vi "Autonomous Independent.vi"() -> ()   [LabVIEW 2017]
doc: "This VI is called when autonomous begins, and will automatically be terminated when autonomous ends. You can carry out timed or sensor driven robot movement independently without needing to return to the caller."
uses:
  <vilib>/Rock Robotics/WPI/DriverStation/WPI_DriverStationRobotMode2.ctl
  <vilib>/Rock Robotics/WPI/ThirdParty/Phoenix-LabVIEW/Motor Controller/Controls/CTRE_Phoenix_MotorControl_ControlMode.ctl
  <vilib>/Rock Robotics/WPI/Utilities/WPI_GetSetVariantRefNum.vi
  <vilib>/Rock Robotics/Network Tables/NT Read String.vi
  <vilib>/Rock Robotics/Network Tables/NT Write Numeric Array.vi
  <vilib>/Rock Robotics/Network Tables/NT Read Number.vi
  <vilib>/Rock Robotics/Network Tables/NT Write String.vi
  Robot Global Data.vi
  <vilib>/Rock Robotics/Network Tables/NT Write Number.vi
  navx-mxp/labview/navX Library v2/navX Library v2.lvlib
panel:
  out "Game Specific Data":string
  # "Be sure to right-click and choose Data Operations>>Make Current Value default if you want to save the array values with the VI"
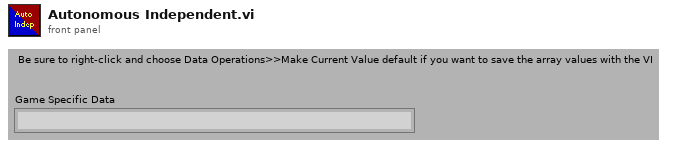
[diagram p1: front panel]
types:
  T1 = typedef "navX Library v2.lvlib/Z900_navX_DeviceTypeDef.ctl" = cluster{"Interface":cluster{"Protocol":T2, "Update Rate (4Hz-100Hz)":u8, "navX Open TypeDef":variant}, "Notify Packet":refnum<notifier>, "Loop VI Refnum":refnum<vi>, "Ready to Close Occurrence Refnum":refnum<k4>}
  T2 = typedef "navX Library v2.lvlib/Z900_navX_ProtocolTypeDef.ctl" = enum16{"SERIAL", "I2C", "SPI"}
  T3 = typedef "WPI_DriverStationRobotMode2.ctl" = enum16{"Autonomous Disabled", "Autonomous Enabled", "Teleop Disabled", "Teleop Enabled", "Disconnected", "Finish", "Test Disabled", "Test Enabled", "Emergency Stopped"}
  T4 = cluster{"Yaw":dbl, "Roll":dbl, "Pitch":dbl, "Heading":dbl, "Fused Heading":dbl}
  T5 = typedef "WPI_GyroDevRef.ctl" = cluster{"DevStatus":errorcluster, "Analog Channel":T6, "Gain (VoltsPerDegree/Second)":dbl, "Gyro Type":enum16{"Analog", "XRS450"}, "Handle":i32, "SPI Bus":T7, "Device Found":bool, "Sample Rate":dbl, "Calibrate On Open":bool, "Offset":dbl}
  T6 = typedef "FPGA_AIChannel.ctl" = enum8{"AI 0", "AI 1", "AI 2", "AI 3", "AI MXP 0", "AI MXP 1", "AI MXP 2", "AI MXP 3", "Invalid"}
  T7 = typedef "spi_bus.ctl" = enum16{"SPI On-Board, CS0", "SPI On-Board, CS1", "SPI On-Board, CS2", "SPI On-Board, CS3", "SPI MXP", "Invalid"}
  T8 = typedef "WPI_JoystickDevRef.ctl" = cluster{"Device":T9}
  T9 = typedef "WPI_JoystickDeviceEnum.ctl" = enum16{"USB 0", "USB 1", "USB 2", "USB 3", "USB 4", "USB 5"}
  T10 = typedef "CTRE_Phoenix_MotorControl_ControlMode.ctl" = u16
  T11 = typedef "WPI_MotorControlDeviceRef.ctl" = cluster{"DeviceStatus":errorcluster, "Type":T12, "PWM":cluster{"PWM Channel":T13, "DeadBand":T14}, "CAN":cluster{"Device Number":u8, "SetOutput VI Ref":variant, "GetOutput VI Ref":variant, "Enable VI Ref":variant, "Disable VI Ref":variant, "Data":variant}, "Invert":bool, "DIO PWM":cluster{"PWM \"Enable\" Channel":T13, "DIOChannel":T15, "PWM Rate":dbl}}
  T12 = typedef "WPI_MotorControlType.ctl" = enum16{"PWM", "CAN", "DIO PWM"}
  T13 = typedef "FPGA_DIOPWMChannel.ctl" = enum8{"PWM 0", "PWM 1", "PWM 2", "PWM 3", "PWM 4", "PWM 5", "PWM 6", "PWM 7", "PWM 8", "PWM 9", "PWM MXP 0", "PWM MXP 1", "PWM MXP 2", "PWM MXP 3", "PWM MXP 4", "PWM MXP 5", "PWM MXP 6", "PWM MXP 7", "PWM MXP 8", "PWM MXP 9", "Invalid"}
  T14 = typedef "WPI_PWMDeadband.ctl" = cluster{"Name":string, "maxPositivePwm":i32, "minPositivePwm":i32, "centerPwm":i32, "maxNegativePwm":i32, "minNegativePwm":i32, "angularRange":u16}
  T15 = typedef "FPGA_DIOChannel.ctl" = enum8{"DIO 0", "DIO 1", "DIO 2", "DIO 3", "DIO 4", "DIO 5", "DIO 6", "DIO 7", "DIO 8", "DIO 9", "DIO MXP 0", "DIO MXP 1", "DIO MXP 2", "DIO MXP 3", "DIO MXP 4", "DIO MXP 5", "DIO MXP 6", "DIO MXP 7", "DIO MXP 8", "DIO MXP 9", "DIO MXP 10", "DIO MXP 11", "DIO MXP 12", "DIO MXP 13", "DIO MXP 14", "DIO MXP 15", "SPI Port CS1", "SPI Port CS2", "SPI Port CS3", "SPI Port MISO", "SPI Port MOSI", "Invalid"}
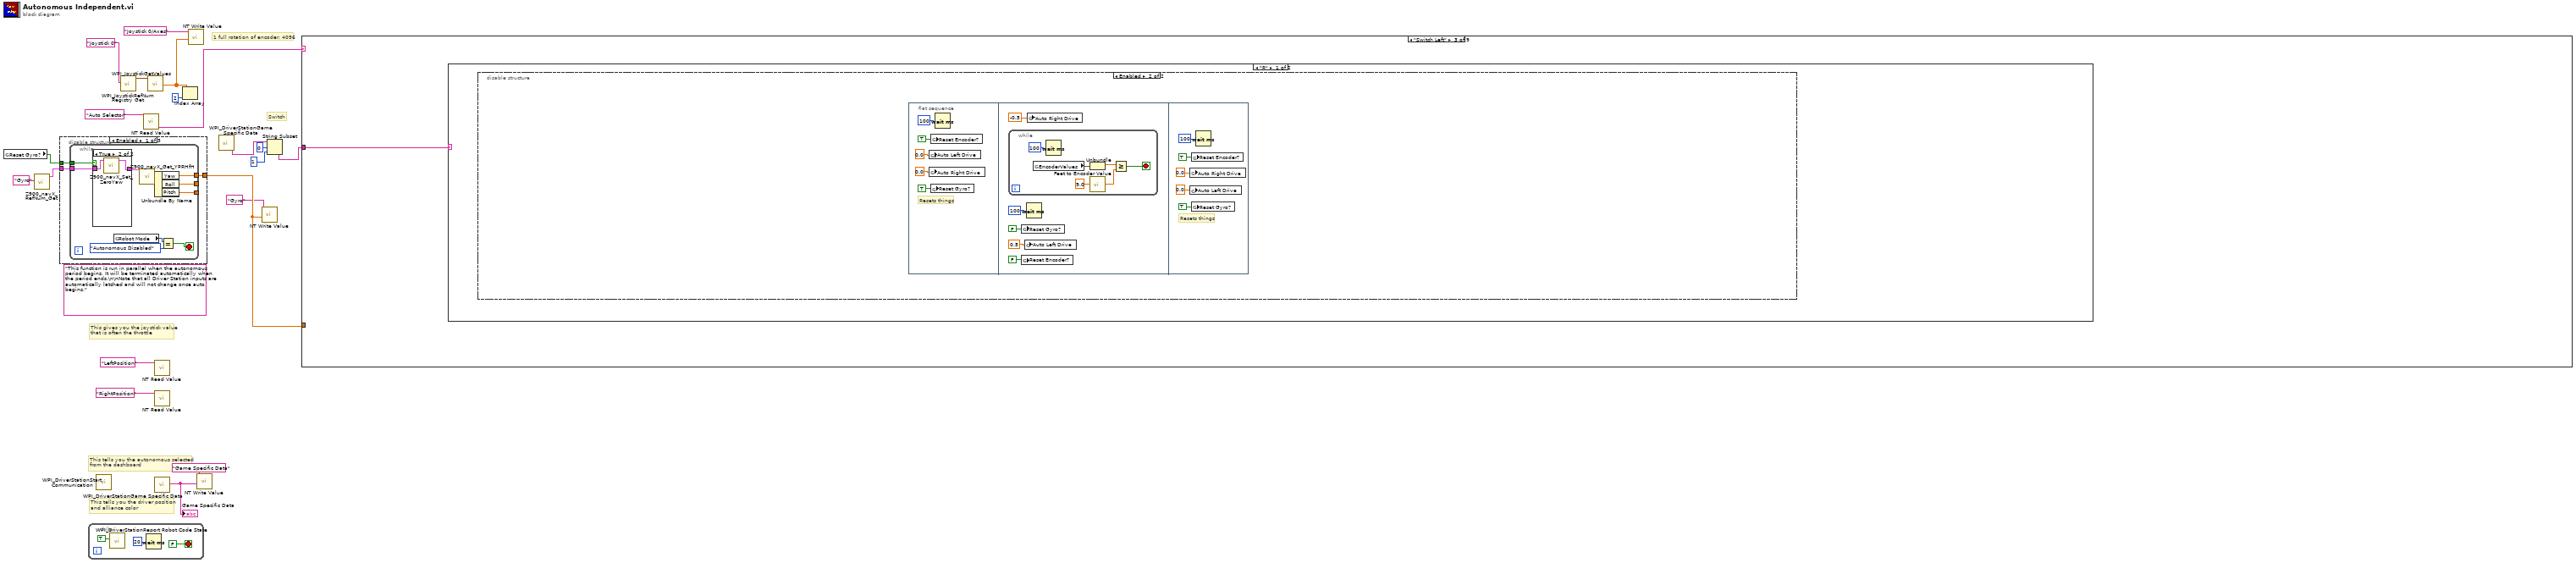
[diagram p0: block diagram]
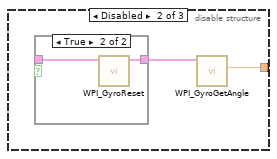
[diagram p3: hidden frame]
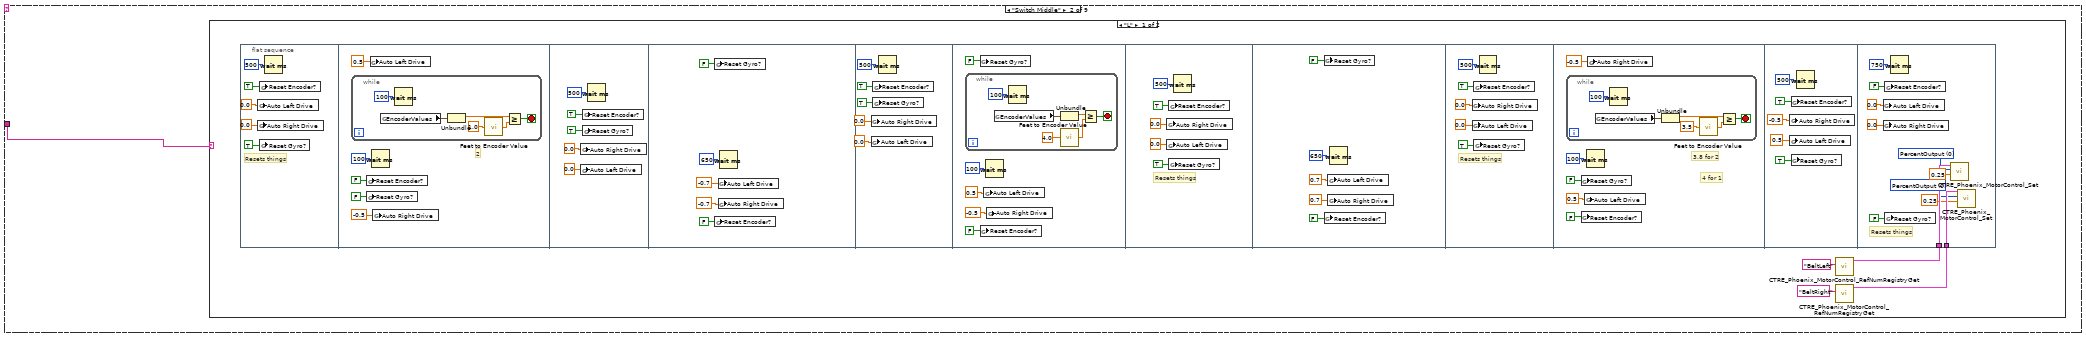
[diagram p7: hidden frame]
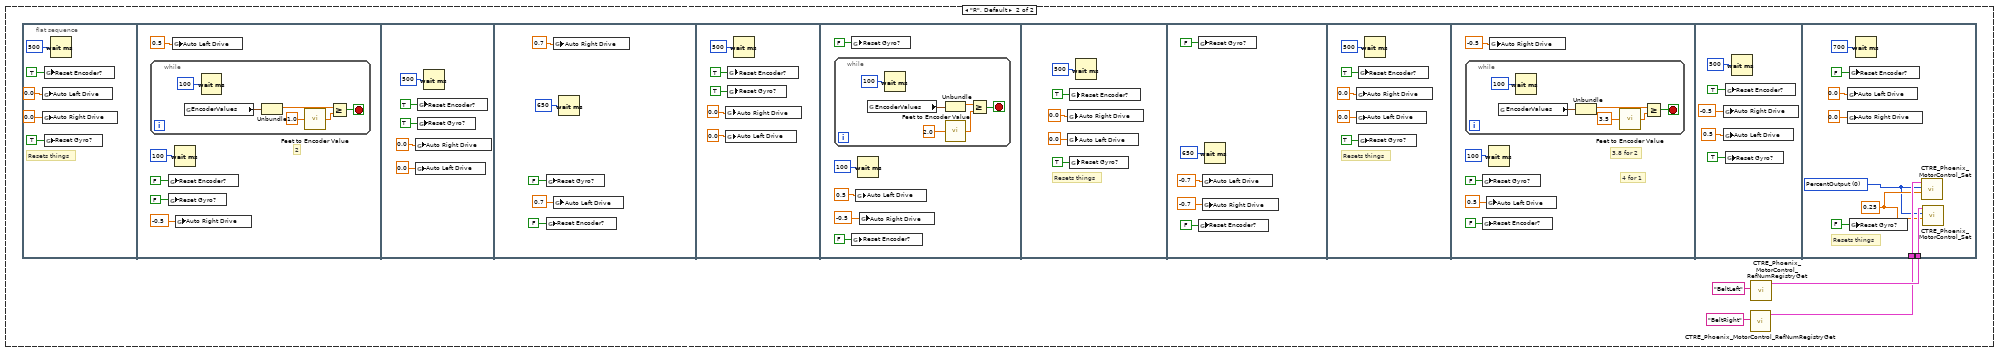
[diagram p8: hidden frame]
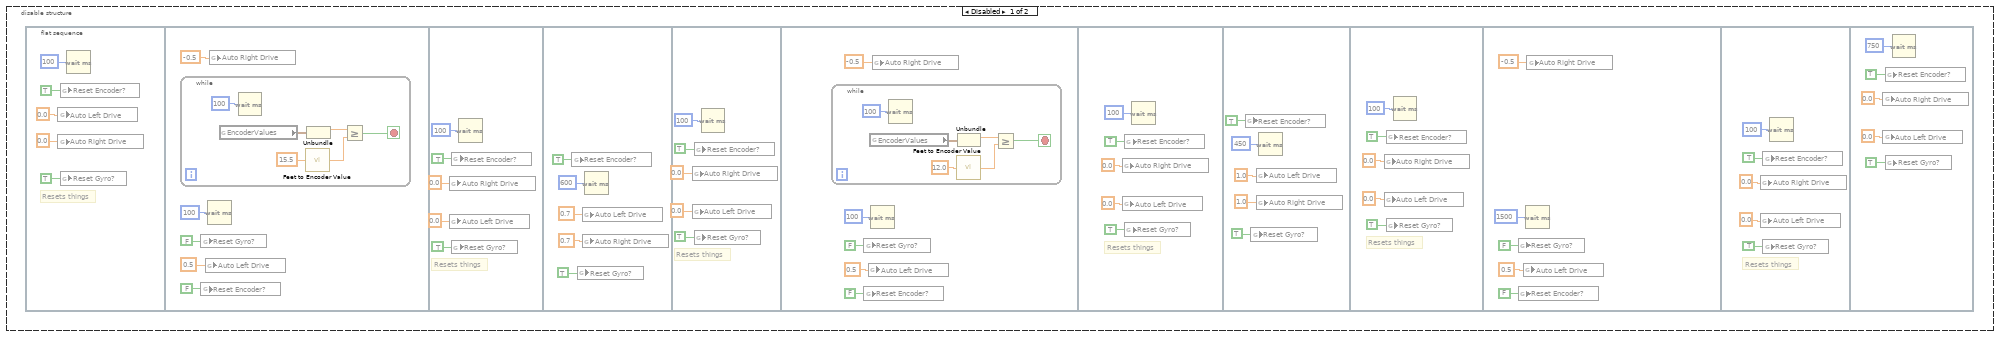
[diagram p9: hidden frame]
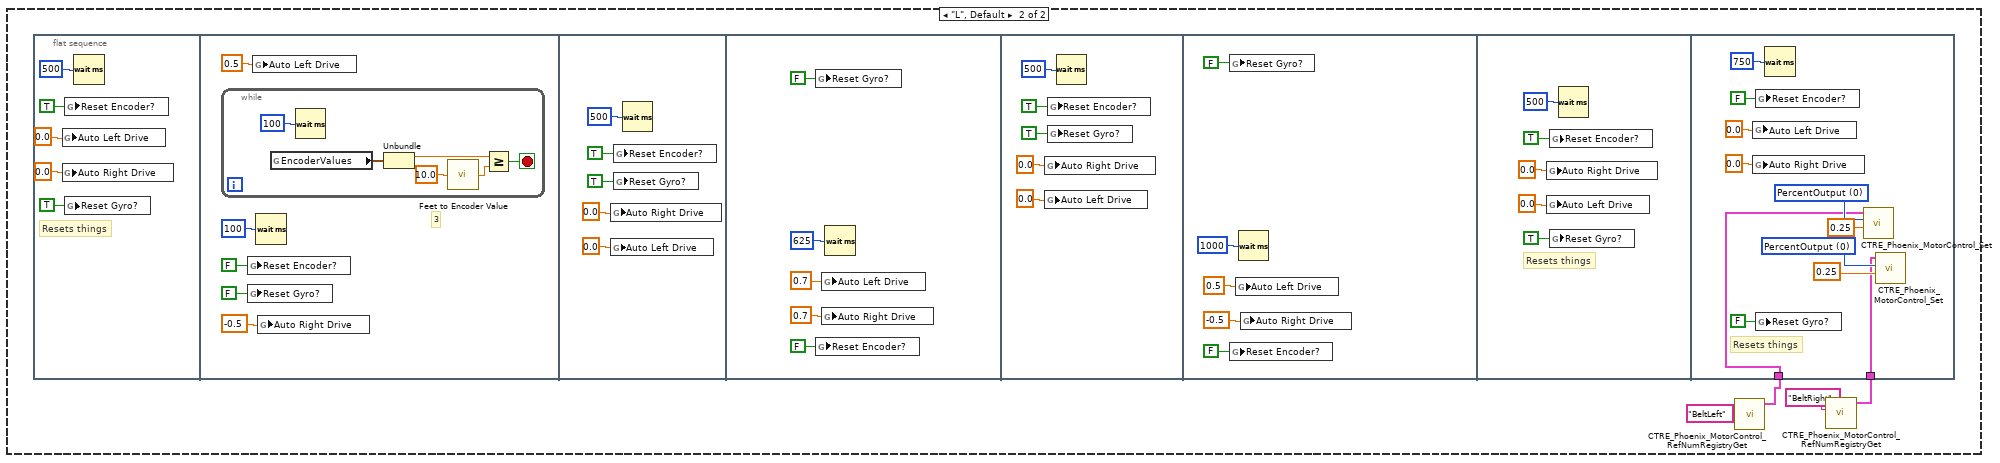
[diagram p10: hidden frame]
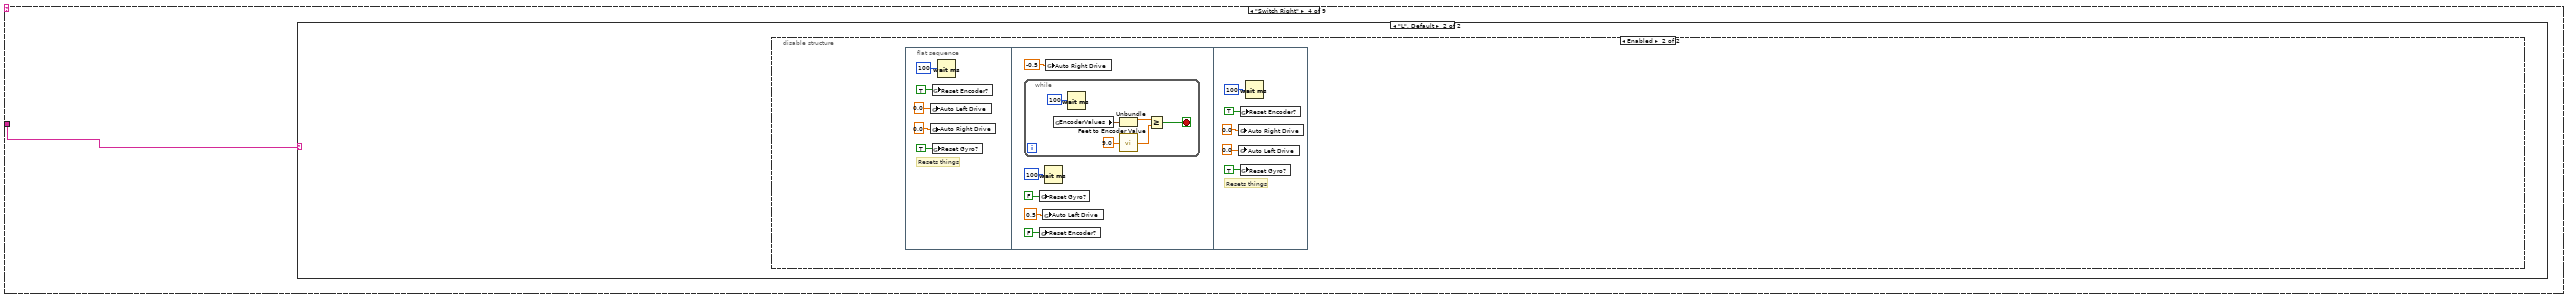
[diagram p11: hidden frame]
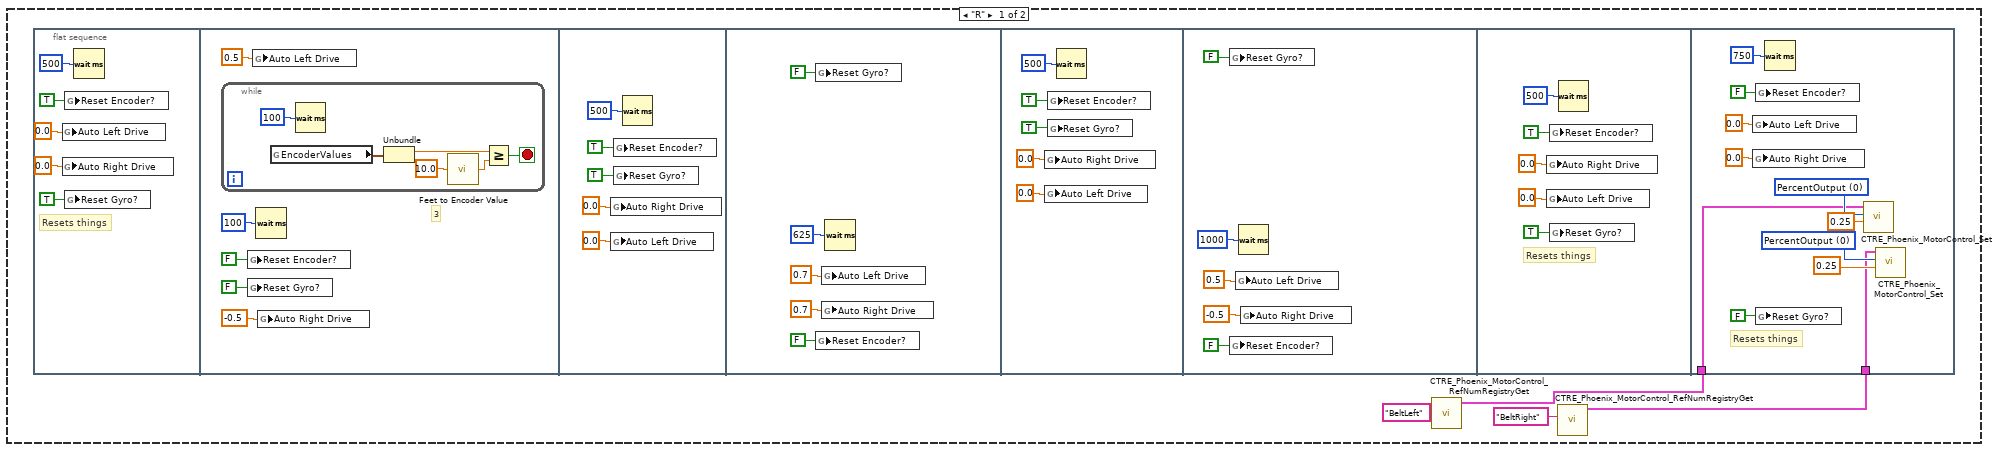
[diagram p12: hidden frame]
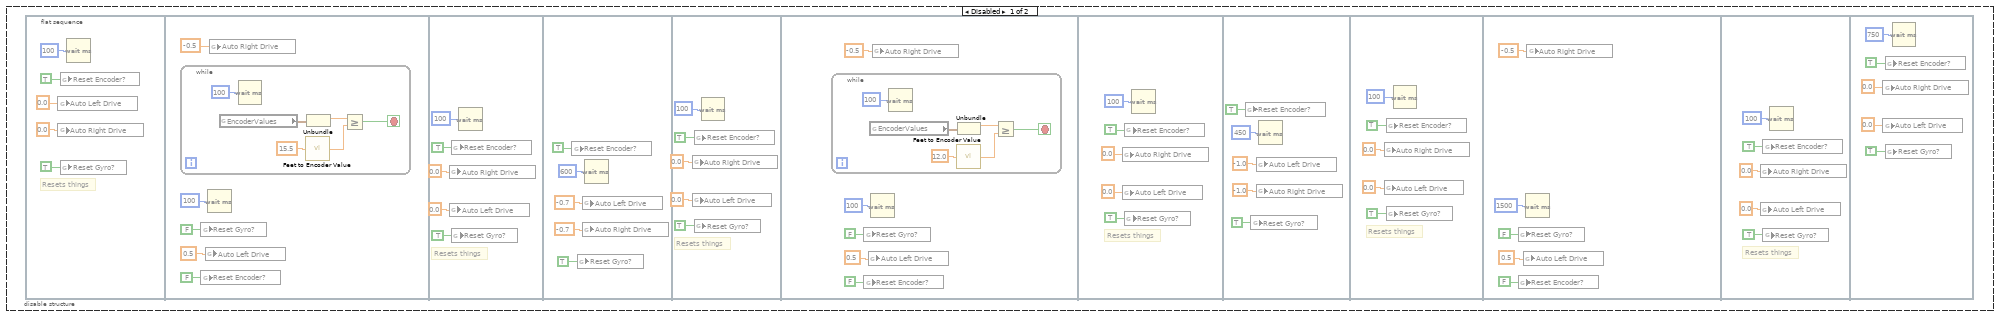
[diagram p13: hidden frame]
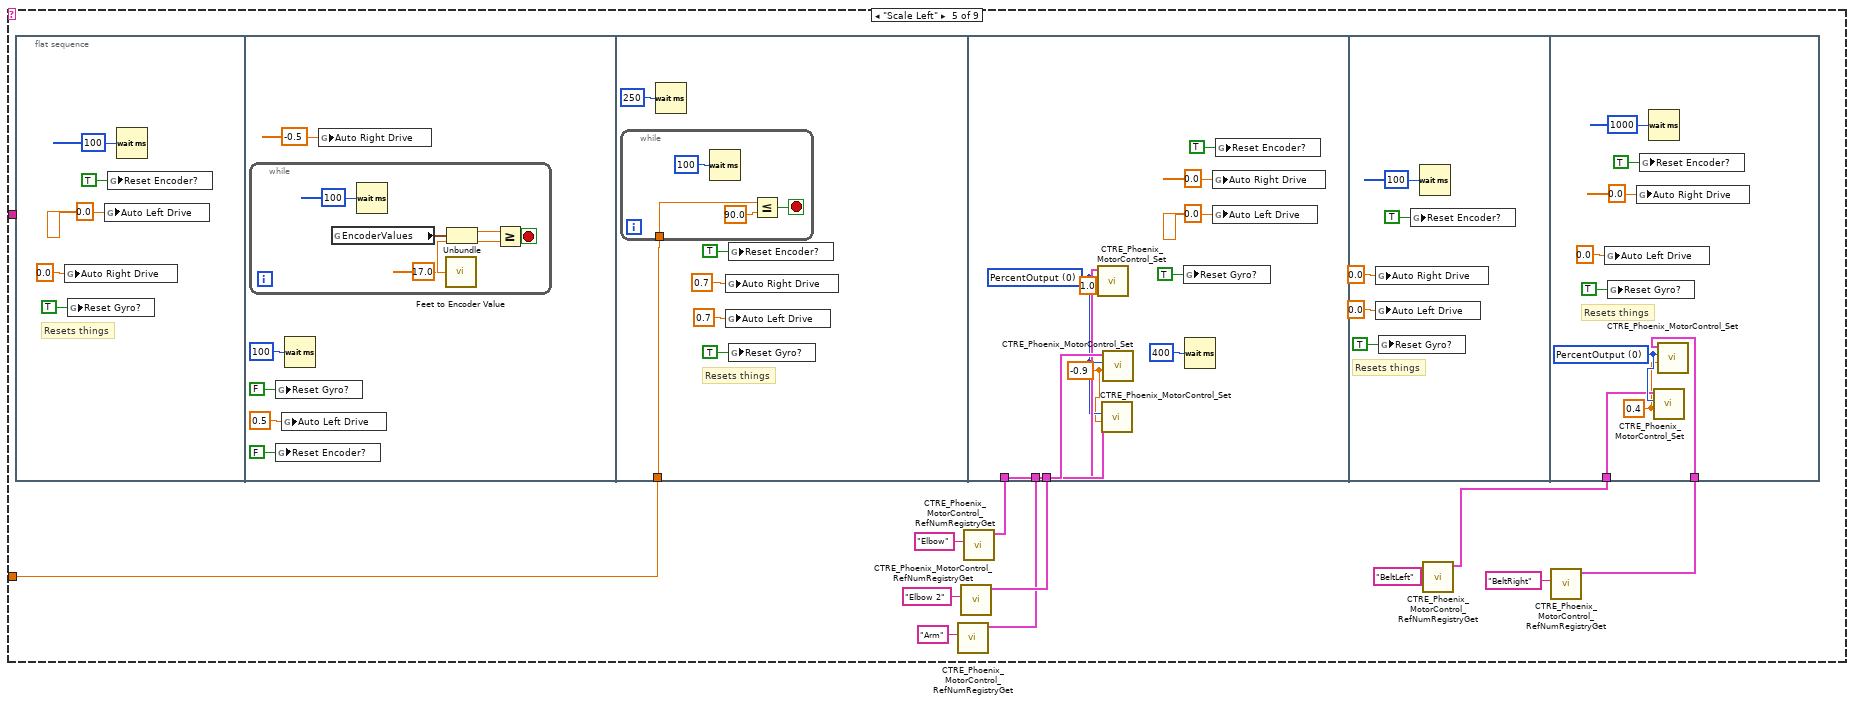
[diagram p14: hidden frame]
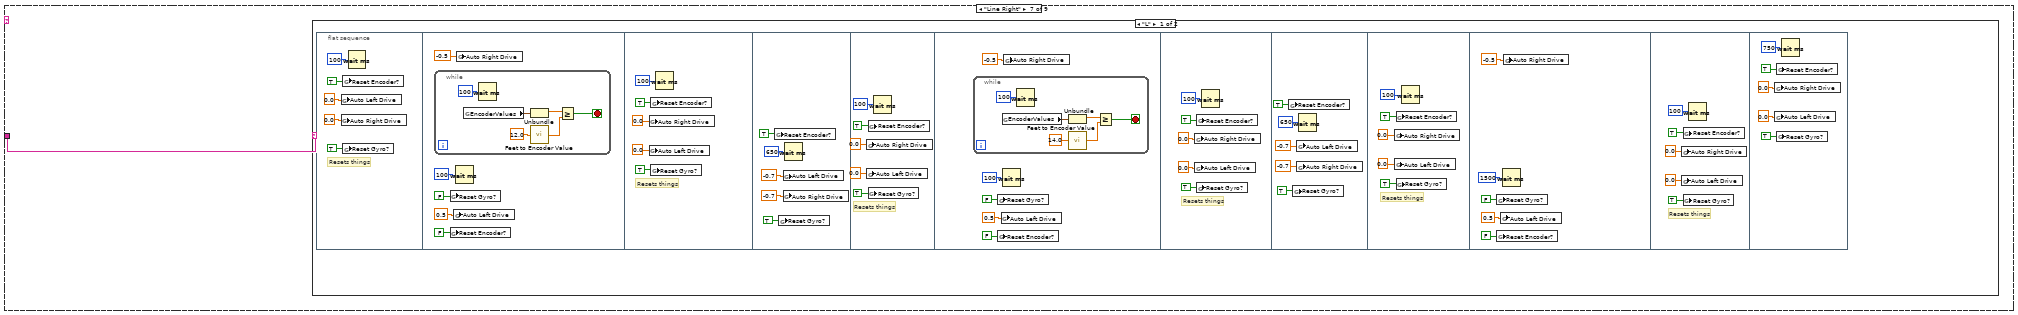
[diagram p16: hidden frame]
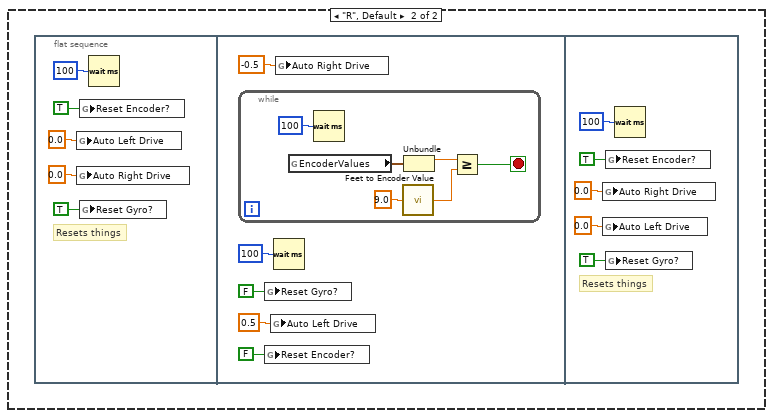
[diagram p17: hidden frame]
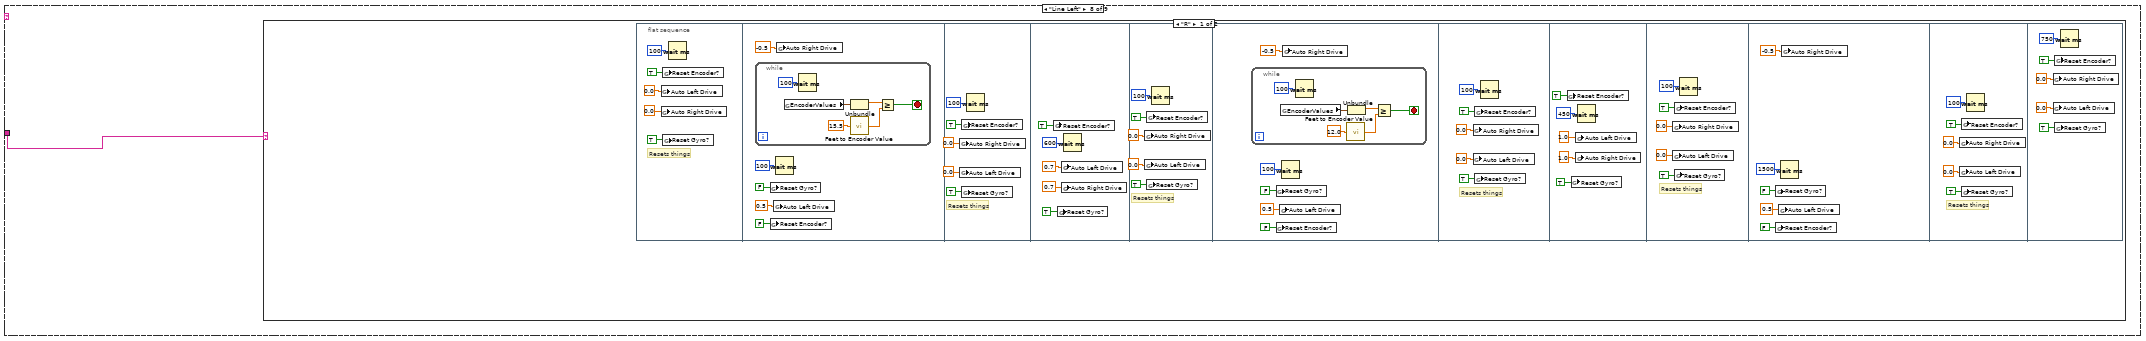
[diagram p18: hidden frame]
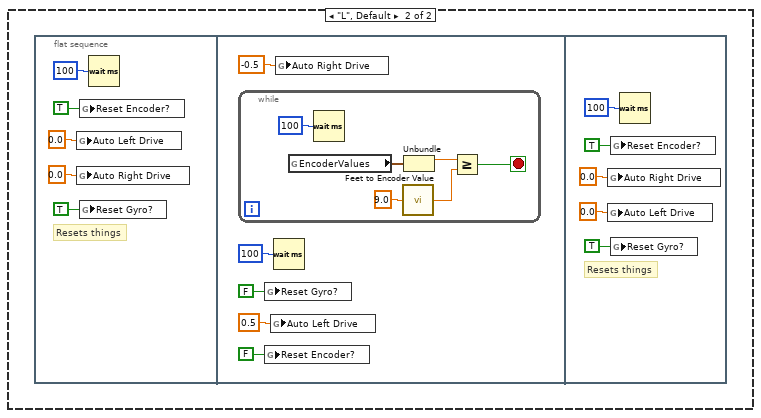
[diagram p19: hidden frame]
diagram:
  (unwired) "This function is run in parallel when the autonomous period begins. It will be terminated automatically when the period ends.\n\nNote that all Driver Station inputs are automatically latched and will not change once auto begins."
  # "Switch"
  # "1 full rotation of encoder: 4096"
  # "This tells you the autonomous selected\nfrom the dashboard"
  # "This gives you the joystick value\nthat is often the throttle"
  # "This tells you the driver position\nand alliance color"
  n1 = global read "Robot Global Data.vi" "Reset Gyro?"() -> (w3:bool)
  n2 = call "Z900_navX_RefNum_Get.vi"("refnum name"="Gyro") -> ("navX Device"=w2:T1)  [unwired: 9 in, 1 out]
  n3 = disable-structure shown="Enabled" {
    disable-tunnel: [w23 w37 _] -> w5
    disable-tunnel: w3 -> [w22 _ _]
    disable-tunnel: w2 -> [w21 _ _]
    frame Enabled {
      n4 = while {
        tunnel: [w27] -> w23
        tunnel: w22 -> [w30]
        tunnel: w21 -> [w26]
        tunnel: [w25] -> _
        tunnel: [w24] -> _
        stop <- w31 stop-if-true
        n5 = case shown="True" w30 {
          tunnel: [w34 w36] -> w29
          tunnel: w26 -> [w34 w35]
          frame False {
          }
          frame True {
            n6 = call "Z900_navX_Set_ZeroYaw.vi"("navX Device"=w35) -> ("navX Device"=w36:T1)  [unwired: 9 in, 1 out]
          }
        }
        n7 = global read "Robot Global Data.vi" "Robot Mode"() -> (w33:T3)
        n8 = call "Z900_navX_Get_YPRHfH.vi"("navX Device"=w29) -> ("YRPHfH"=w28:T4)  [unwired: 7 in, 3 out]
        n9 = Unbundle By Name(w28) -> ("Yaw"=w27:dbl, "Roll"=w25:dbl, "Pitch"=w24:dbl)
        n10 = Equal?(x=w33, y=WPI_DriverStationRobotMode2."Autonomous Disabled") -> (x = y?=w31:bool)
      }
    }
    frame Disabled {
      n11 = case shown="True" {
        selector: _ -> [_ _]
        tunnel: _ -> [w39 w41]
        tunnel: [w39 w40] -> w38
        frame False {
        }
        frame True {
          n12 = call <vilib>:"WPI_GyroReset.vi"("GyroDevRef"=w41) -> ("GyroDevRef"=w40:T5)  [unwired: 9 in, 1 out]
        }
      }
      n13 = call <vilib>:"WPI_GyroGetAngle.vi"("GyroDevRef"=w38) -> ("Angle"=w37:dbl)  [unwired: 6 in, 4 out]
    }
    frame Disabled {
      # "Everything is off :("
    }
  }
  n14 = while {
    stop <- FALSE stop-if-true
    n15 = call <vilib>:"WPI_DriverStationReport Robot Code State.vi"("Autonomous"=TRUE) -> ()  [unwired: 10 in, 1 out]
    n16 = Wait (ms)(milliseconds to wait=u32 20) -> ()  [unwired: 1 out]
  }
  n17 = call <vilib>:"WPI_DriverStationStart Communication.vi"() -> ()  [unwired: 12 in]
  n18 = call <vilib>:"WPI_JoystickRefNum Registry Get.vi"("refnum name"="Joystick 0") -> ("JoystickDevRef"=w19:T8)  [unwired: 1 in, 9 out]
  n19 = call-poly <vilib>:"NT Read Value.vi"("Name"="Auto Selector") -> ("String"=w17:string)  [unwired: 9 in, 1 out]
  n20 = call <vilib>:"WPI_JoystickGetValues.vi"("JoystickDevRef"=w19) -> ("Axes"=w16:dbl[])  [unwired: 6 in, 4 out]
  n21 = call-poly <vilib>:"NT Read Value.vi"("Name"="RightPosition") -> ()  [unwired: 9 in, 2 out]
  n22 = call <vilib>:"WPI_DriverStationGame Specific Data.vi"() -> ("Game Specific Data"=w12:string)  [unwired: 11 in]
  "Game Specific Data" <- w12
  n23 = call-poly <vilib>:"NT Read Value.vi"("Name"="LeftPosition") -> ()  [unwired: 9 in, 2 out]
  n24 = Index Array(array=w16, index=2) -> ()  [unwired: 1 out]
  n25 = call-poly <vilib>:"NT Write Value.vi"("Numeric Array"=w16, "Name"="Joystick 0/Axes") -> ()  [unwired: 9 in, 1 out]
  n26 = call-poly <vilib>:"NT Write Value.vi"("String"=w12, "Name"="Game Specific Data") -> ()  [unwired: 9 in, 1 out]
  n27 = call <vilib>:"WPI_DriverStationGame Specific Data.vi"() -> ("Game Specific Data"=w7:string)  [unwired: 11 in]
  n28 = call-poly <vilib>:"NT Write Value.vi"("Numeric"=w5, "Name"="Gyro") -> ()  [unwired: 9 in, 1 out]
  n29 = String Subset(string=w7, offset (0)=0, length (rest)=1 ("length (rest)")) -> (substring=w8:string)
  n30 = case shown="\"Switch Left\"" w17 {
    tunnel: w8 -> [_ w45 w220 w370 _ _ w581 w675 _]
    tunnel: w5 -> [_ _ _ _ w520 _ _ _ _]
    frame Default {
      # "You can put your main auto here, or you can right-click on the case and make any\nother frame be the default case."
      # "This is the frame that will execute if no selection is made, or if it is not recognized"
    }
    frame "Switch Middle" {
      n31 = case shown="\"L\"" w45 {
        frame "L" {
          n32 = flat-sequence {
            tunnel: w47 -> [w128]
            tunnel: w46 -> [w127]
            frame #0 {
              # "Resets things"
              n33 = global write "Robot Global Data.vi" "Auto Left Drive"(0.0 ("Auto Left Drive")) -> ()
              n34 = global write "Robot Global Data.vi" "Auto Right Drive"(0.0 ("Auto Right Drive")) -> ()
              n35 = global write "Robot Global Data.vi" "Reset Encoder?"(TRUE ("Reset Encoder?")) -> ()
              n36 = global write "Robot Global Data.vi" "Reset Gyro?"(TRUE ("Reset Gyro?")) -> ()
              n37 = Wait (ms)(milliseconds to wait=u32 500) -> ()  [unwired: 1 out]
            }
            frame #1 {
              # "2"
              n38 = while {
                stop <- w60 stop-if-true
                n39 = global read "Robot Global Data.vi" "EncoderValues"() -> (w65:cluster{"EncoderLeft":dbl, "EncoderRight":dbl})
                n40 = Wait (ms)(milliseconds to wait=u32 100) -> ()  [unwired: 1 out]
                n41 = Unbundle(w65) -> ("EncoderLeft"=w64:dbl)  [unwired: 1 out]
                n42 = call "Feet to Encoder Value.vi"("Feet"=1.0) -> ("Encoder Value"=w63:dbl)
                n43 = Greater Or Equal?(x=w64, y=w63) -> (x >= y?=w60:bool)
              }
              n44 = global write "Robot Global Data.vi" "Reset Encoder?"(FALSE ("Reset Encoder?")) -> ()
              n45 = global write "Robot Global Data.vi" "Reset Gyro?"(FALSE ("Reset Gyro?")) -> ()
              n46 = global write "Robot Global Data.vi" "Auto Left Drive"(0.5 ("Auto Left Drive")) -> ()
              n47 = Wait (ms)(milliseconds to wait=u32 100) -> ()  [unwired: 1 out]
              n48 = global write "Robot Global Data.vi" "Auto Right Drive"(-0.5 ("Auto Right Drive")) -> ()
            }
            frame #2 {
              n49 = global write "Robot Global Data.vi" "Auto Right Drive"(0.0 ("Auto Right Drive")) -> ()
              n50 = global write "Robot Global Data.vi" "Auto Left Drive"(0.0 ("Auto Left Drive")) -> ()
              n51 = global write "Robot Global Data.vi" "Reset Encoder?"(TRUE ("Reset Encoder?")) -> ()
              n52 = global write "Robot Global Data.vi" "Reset Gyro?"(TRUE ("Reset Gyro?")) -> ()
              n53 = Wait (ms)(milliseconds to wait=u32 500) -> ()  [unwired: 1 out]
            }
            frame #3 {
              n54 = global write "Robot Global Data.vi" "Reset Gyro?"(FALSE ("Reset Gyro?")) -> ()
              n55 = global write "Robot Global Data.vi" "Reset Encoder?"(FALSE ("Reset Encoder?")) -> ()
              n56 = global write "Robot Global Data.vi" "Auto Left Drive"(-0.7 ("Auto Left Drive")) -> ()
              n57 = global write "Robot Global Data.vi" "Auto Right Drive"(-0.7 ("Auto Right Drive")) -> ()
              n58 = Wait (ms)(milliseconds to wait=u32 650) -> ()  [unwired: 1 out]
            }
            frame #4 {
              n59 = global write "Robot Global Data.vi" "Auto Right Drive"(0.0 ("Auto Right Drive")) -> ()
              n60 = global write "Robot Global Data.vi" "Auto Left Drive"(0.0 ("Auto Left Drive")) -> ()
              n61 = global write "Robot Global Data.vi" "Reset Encoder?"(TRUE ("Reset Encoder?")) -> ()
              n62 = global write "Robot Global Data.vi" "Reset Gyro?"(TRUE ("Reset Gyro?")) -> ()
              n63 = Wait (ms)(milliseconds to wait=u32 500) -> ()  [unwired: 1 out]
            }
            frame #5 {
              n64 = while {
                stop <- w86 stop-if-true
                n65 = global read "Robot Global Data.vi" "EncoderValues"() -> (w91:cluster{"EncoderLeft":dbl, "EncoderRight":dbl})
                n66 = Wait (ms)(milliseconds to wait=u32 100) -> ()  [unwired: 1 out]
                n67 = Unbundle(w91) -> ("EncoderLeft"=w90:dbl)  [unwired: 1 out]
                n68 = call "Feet to Encoder Value.vi"("Feet"=4.0) -> ("Encoder Value"=w89:dbl)
                n69 = Greater Or Equal?(x=w90, y=w89) -> (x >= y?=w86:bool)
              }
              n70 = global write "Robot Global Data.vi" "Reset Gyro?"(FALSE ("Reset Gyro?")) -> ()
              n71 = global write "Robot Global Data.vi" "Reset Encoder?"(FALSE ("Reset Encoder?")) -> ()
              n72 = global write "Robot Global Data.vi" "Auto Left Drive"(0.5 ("Auto Left Drive")) -> ()
              n73 = Wait (ms)(milliseconds to wait=u32 100) -> ()  [unwired: 1 out]
              n74 = global write "Robot Global Data.vi" "Auto Right Drive"(-0.5 ("Auto Right Drive")) -> ()
            }
            frame #6 {
              # "Resets things"
              n75 = global write "Robot Global Data.vi" "Auto Right Drive"(0.0 ("Auto Right Drive")) -> ()
              n76 = global write "Robot Global Data.vi" "Auto Left Drive"(0.0 ("Auto Left Drive")) -> ()
              n77 = global write "Robot Global Data.vi" "Reset Encoder?"(TRUE ("Reset Encoder?")) -> ()
              n78 = global write "Robot Global Data.vi" "Reset Gyro?"(TRUE ("Reset Gyro?")) -> ()
              n79 = Wait (ms)(milliseconds to wait=u32 500) -> ()  [unwired: 1 out]
            }
            frame #7 {
              n80 = global write "Robot Global Data.vi" "Reset Gyro?"(FALSE ("Reset Gyro?")) -> ()
              n81 = global write "Robot Global Data.vi" "Reset Encoder?"(FALSE ("Reset Encoder?")) -> ()
              n82 = global write "Robot Global Data.vi" "Auto Left Drive"(0.7 ("Auto Left Drive")) -> ()
              n83 = global write "Robot Global Data.vi" "Auto Right Drive"(0.7 ("Auto Right Drive")) -> ()
              n84 = Wait (ms)(milliseconds to wait=u32 650) -> ()  [unwired: 1 out]
            }
            frame #8 {
              # "Resets things"
              n85 = global write "Robot Global Data.vi" "Auto Right Drive"(0.0 ("Auto Right Drive")) -> ()
              n86 = global write "Robot Global Data.vi" "Auto Left Drive"(0.0 ("Auto Left Drive")) -> ()
              n87 = global write "Robot Global Data.vi" "Reset Encoder?"(TRUE ("Reset Encoder?")) -> ()
              n88 = global write "Robot Global Data.vi" "Reset Gyro?"(TRUE ("Reset Gyro?")) -> ()
              n89 = Wait (ms)(milliseconds to wait=u32 500) -> ()  [unwired: 1 out]
            }
            frame #9 {
              # "4 for 1"
              # "3.8 for 2"
              n90 = while {
                stop <- w112 stop-if-true
                n91 = global read "Robot Global Data.vi" "EncoderValues"() -> (w117:cluster{"EncoderLeft":dbl, "EncoderRight":dbl})
                n92 = Wait (ms)(milliseconds to wait=u32 100) -> ()  [unwired: 1 out]
                n93 = Unbundle(w117) -> ("EncoderLeft"=w116:dbl)  [unwired: 1 out]
                n94 = call "Feet to Encoder Value.vi"("Feet"=3.5) -> ("Encoder Value"=w115:dbl)
                n95 = Greater Or Equal?(x=w116, y=w115) -> (x >= y?=w112:bool)
              }
              n96 = global write "Robot Global Data.vi" "Reset Gyro?"(FALSE ("Reset Gyro?")) -> ()
              n97 = global write "Robot Global Data.vi" "Reset Encoder?"(FALSE ("Reset Encoder?")) -> ()
              n98 = global write "Robot Global Data.vi" "Auto Left Drive"(0.5 ("Auto Left Drive")) -> ()
              n99 = Wait (ms)(milliseconds to wait=u32 100) -> ()  [unwired: 1 out]
              n100 = global write "Robot Global Data.vi" "Auto Right Drive"(-0.5 ("Auto Right Drive")) -> ()
            }
            frame #10 {
              n101 = global write "Robot Global Data.vi" "Auto Right Drive"(-0.5 ("Auto Right Drive")) -> ()
              n102 = global write "Robot Global Data.vi" "Auto Left Drive"(0.5 ("Auto Left Drive")) -> ()
              n103 = global write "Robot Global Data.vi" "Reset Encoder?"(TRUE ("Reset Encoder?")) -> ()
              n104 = global write "Robot Global Data.vi" "Reset Gyro?"(TRUE ("Reset Gyro?")) -> ()
              n105 = Wait (ms)(milliseconds to wait=u32 500) -> ()  [unwired: 1 out]
            }
            frame #11 {
              w125 = T10 0 items=["PercentOutput"=0, "Position"=1, "Velocity"=2, "Current"=3, "Follower"=5, "MotionProfile"=6, "MotionMagic"=7, "MotionMagicArc"=8, "MotionProfileArc"=10, "Disabled"=15] ("Control Mode")
              w126 = T10 0 items=["PercentOutput"=0, "Position"=1, "Velocity"=2, "Current"=3, "Follower"=5, "MotionProfile"=6, "MotionMagic"=7, "MotionMagicArc"=8, "MotionProfileArc"=10, "Disabled"=15] ("Control Mode")
              # "Resets things"
              n106 = global write "Robot Global Data.vi" "Auto Left Drive"(0.0 ("Auto Left Drive")) -> ()
              n107 = global write "Robot Global Data.vi" "Auto Right Drive"(0.0 ("Auto Right Drive")) -> ()
              n108 = global write "Robot Global Data.vi" "Reset Encoder?"(FALSE ("Reset Encoder?")) -> ()
              n109 = global write "Robot Global Data.vi" "Reset Gyro?"(FALSE ("Reset Gyro?")) -> ()
              n110 = Wait (ms)(milliseconds to wait=u32 750) -> ()  [unwired: 1 out]
              n111 = call <vilib>:"CTRE_Phoenix_MotorControl_Set.vi"("Output"=0.25, "Control Mode"=w126, "PhoenixMotorControlDevRef"=w128) -> ()  [unwired: 7 in, 2 out]
              n112 = call <vilib>:"CTRE_Phoenix_MotorControl_Set.vi"("Output"=0.25, "Control Mode"=w125, "PhoenixMotorControlDevRef"=w127) -> ()  [unwired: 7 in, 2 out]
            }
          }
          n113 = call <vilib>:"CTRE_Phoenix_MotorControl_RefNumRegistryGet.vi"("refnum name"="BeltRight") -> ("PhoenixMotorControlDevRef"=w46:T11)  [unwired: 9 in, 1 out]
          n114 = call <vilib>:"CTRE_Phoenix_MotorControl_RefNumRegistryGet.vi"("refnum name"="BeltLeft") -> ("PhoenixMotorControlDevRef"=w47:T11)  [unwired: 9 in, 1 out]
        }
        frame "R", Default {
          n115 = flat-sequence {
            tunnel: w135 -> [w214]
            tunnel: w134 -> [w213]
            frame #0 {
              # "Resets things"
              n116 = global write "Robot Global Data.vi" "Auto Left Drive"(0.0 ("Auto Left Drive")) -> ()
              n117 = global write "Robot Global Data.vi" "Auto Right Drive"(0.0 ("Auto Right Drive")) -> ()
              n118 = global write "Robot Global Data.vi" "Reset Encoder?"(TRUE ("Reset Encoder?")) -> ()
              n119 = global write "Robot Global Data.vi" "Reset Gyro?"(TRUE ("Reset Gyro?")) -> ()
              n120 = Wait (ms)(milliseconds to wait=u32 500) -> ()  [unwired: 1 out]
            }
            frame #1 {
              # "2"
              n121 = while {
                stop <- w148 stop-if-true
                n122 = global read "Robot Global Data.vi" "EncoderValues"() -> (w153:cluster{"EncoderLeft":dbl, "EncoderRight":dbl})
                n123 = Wait (ms)(milliseconds to wait=u32 100) -> ()  [unwired: 1 out]
                n124 = Unbundle(w153) -> ("EncoderLeft"=w152:dbl)  [unwired: 1 out]
                n125 = call "Feet to Encoder Value.vi"("Feet"=1.0) -> ("Encoder Value"=w151:dbl)
                n126 = Greater Or Equal?(x=w152, y=w151) -> (x >= y?=w148:bool)
              }
              n127 = global write "Robot Global Data.vi" "Reset Encoder?"(FALSE ("Reset Encoder?")) -> ()
              n128 = global write "Robot Global Data.vi" "Reset Gyro?"(FALSE ("Reset Gyro?")) -> ()
              n129 = global write "Robot Global Data.vi" "Auto Left Drive"(0.5 ("Auto Left Drive")) -> ()
              n130 = Wait (ms)(milliseconds to wait=u32 100) -> ()  [unwired: 1 out]
              n131 = global write "Robot Global Data.vi" "Auto Right Drive"(-0.5 ("Auto Right Drive")) -> ()
            }
            frame #2 {
              n132 = global write "Robot Global Data.vi" "Auto Right Drive"(0.0 ("Auto Right Drive")) -> ()
              n133 = global write "Robot Global Data.vi" "Auto Left Drive"(0.0 ("Auto Left Drive")) -> ()
              n134 = global write "Robot Global Data.vi" "Reset Encoder?"(TRUE ("Reset Encoder?")) -> ()
              n135 = global write "Robot Global Data.vi" "Reset Gyro?"(TRUE ("Reset Gyro?")) -> ()
              n136 = Wait (ms)(milliseconds to wait=u32 500) -> ()  [unwired: 1 out]
            }
            frame #3 {
              n137 = global write "Robot Global Data.vi" "Reset Gyro?"(FALSE ("Reset Gyro?")) -> ()
              n138 = global write "Robot Global Data.vi" "Reset Encoder?"(FALSE ("Reset Encoder?")) -> ()
              n139 = global write "Robot Global Data.vi" "Auto Right Drive"(0.7 ("Auto Right Drive")) -> ()
              n140 = global write "Robot Global Data.vi" "Auto Left Drive"(0.7 ("Auto Left Drive")) -> ()
              n141 = Wait (ms)(milliseconds to wait=u32 650) -> ()  [unwired: 1 out]
            }
            frame #4 {
              n142 = global write "Robot Global Data.vi" "Auto Right Drive"(0.0 ("Auto Right Drive")) -> ()
              n143 = global write "Robot Global Data.vi" "Auto Left Drive"(0.0 ("Auto Left Drive")) -> ()
              n144 = global write "Robot Global Data.vi" "Reset Encoder?"(TRUE ("Reset Encoder?")) -> ()
              n145 = global write "Robot Global Data.vi" "Reset Gyro?"(TRUE ("Reset Gyro?")) -> ()
              n146 = Wait (ms)(milliseconds to wait=u32 500) -> ()  [unwired: 1 out]
            }
            frame #5 {
              n147 = while {
                stop <- w174 stop-if-true
                n148 = global read "Robot Global Data.vi" "EncoderValues"() -> (w179:cluster{"EncoderLeft":dbl, "EncoderRight":dbl})
                n149 = Wait (ms)(milliseconds to wait=u32 100) -> ()  [unwired: 1 out]
                n150 = Unbundle(w179) -> ("EncoderLeft"=w178:dbl)  [unwired: 1 out]
                n151 = call "Feet to Encoder Value.vi"("Feet"=2.0) -> ("Encoder Value"=w177:dbl)
                n152 = Greater Or Equal?(x=w178, y=w177) -> (x >= y?=w174:bool)
              }
              n153 = global write "Robot Global Data.vi" "Reset Gyro?"(FALSE ("Reset Gyro?")) -> ()
              n154 = global write "Robot Global Data.vi" "Reset Encoder?"(FALSE ("Reset Encoder?")) -> ()
              n155 = global write "Robot Global Data.vi" "Auto Left Drive"(0.5 ("Auto Left Drive")) -> ()
              n156 = Wait (ms)(milliseconds to wait=u32 100) -> ()  [unwired: 1 out]
              n157 = global write "Robot Global Data.vi" "Auto Right Drive"(-0.5 ("Auto Right Drive")) -> ()
            }
            frame #6 {
              # "Resets things"
              n158 = global write "Robot Global Data.vi" "Auto Right Drive"(0.0 ("Auto Right Drive")) -> ()
              n159 = global write "Robot Global Data.vi" "Auto Left Drive"(0.0 ("Auto Left Drive")) -> ()
              n160 = global write "Robot Global Data.vi" "Reset Encoder?"(TRUE ("Reset Encoder?")) -> ()
              n161 = global write "Robot Global Data.vi" "Reset Gyro?"(TRUE ("Reset Gyro?")) -> ()
              n162 = Wait (ms)(milliseconds to wait=u32 500) -> ()  [unwired: 1 out]
            }
            frame #7 {
              n163 = global write "Robot Global Data.vi" "Reset Gyro?"(FALSE ("Reset Gyro?")) -> ()
              n164 = global write "Robot Global Data.vi" "Reset Encoder?"(FALSE ("Reset Encoder?")) -> ()
              n165 = global write "Robot Global Data.vi" "Auto Left Drive"(-0.7 ("Auto Left Drive")) -> ()
              n166 = global write "Robot Global Data.vi" "Auto Right Drive"(-0.7 ("Auto Right Drive")) -> ()
              n167 = Wait (ms)(milliseconds to wait=u32 650) -> ()  [unwired: 1 out]
            }
            frame #8 {
              # "Resets things"
              n168 = global write "Robot Global Data.vi" "Auto Right Drive"(0.0 ("Auto Right Drive")) -> ()
              n169 = global write "Robot Global Data.vi" "Auto Left Drive"(0.0 ("Auto Left Drive")) -> ()
              n170 = global write "Robot Global Data.vi" "Reset Encoder?"(TRUE ("Reset Encoder?")) -> ()
              n171 = global write "Robot Global Data.vi" "Reset Gyro?"(TRUE ("Reset Gyro?")) -> ()
              n172 = Wait (ms)(milliseconds to wait=u32 500) -> ()  [unwired: 1 out]
            }
            frame #9 {
              # "4 for 1"
              # "3.8 for 2"
              n173 = while {
                stop <- w200 stop-if-true
                n174 = global read "Robot Global Data.vi" "EncoderValues"() -> (w205:cluster{"EncoderLeft":dbl, "EncoderRight":dbl})
                n175 = Wait (ms)(milliseconds to wait=u32 100) -> ()  [unwired: 1 out]
                n176 = Unbundle(w205) -> ("EncoderLeft"=w204:dbl)  [unwired: 1 out]
                n177 = call "Feet to Encoder Value.vi"("Feet"=3.5) -> ("Encoder Value"=w203:dbl)
                n178 = Greater Or Equal?(x=w204, y=w203) -> (x >= y?=w200:bool)
              }
              n179 = global write "Robot Global Data.vi" "Reset Gyro?"(FALSE ("Reset Gyro?")) -> ()
              n180 = global write "Robot Global Data.vi" "Reset Encoder?"(FALSE ("Reset Encoder?")) -> ()
              n181 = global write "Robot Global Data.vi" "Auto Left Drive"(0.5 ("Auto Left Drive")) -> ()
              n182 = Wait (ms)(milliseconds to wait=u32 100) -> ()  [unwired: 1 out]
              n183 = global write "Robot Global Data.vi" "Auto Right Drive"(-0.5 ("Auto Right Drive")) -> ()
            }
            frame #10 {
              n184 = global write "Robot Global Data.vi" "Auto Right Drive"(-0.5 ("Auto Right Drive")) -> ()
              n185 = global write "Robot Global Data.vi" "Auto Left Drive"(0.5 ("Auto Left Drive")) -> ()
              n186 = global write "Robot Global Data.vi" "Reset Encoder?"(TRUE ("Reset Encoder?")) -> ()
              n187 = global write "Robot Global Data.vi" "Reset Gyro?"(TRUE ("Reset Gyro?")) -> ()
              n188 = Wait (ms)(milliseconds to wait=u32 500) -> ()  [unwired: 1 out]
            }
            frame #11 {
              w211 = T10 0 items=["PercentOutput"=0, "Position"=1, "Velocity"=2, "Current"=3, "Follower"=5, "MotionProfile"=6, "MotionMagic"=7, "MotionMagicArc"=8, "MotionProfileArc"=10, "Disabled"=15] ("Control Mode")
              w212 = 0.25 ("Output")
              # "Resets things"
              n189 = global write "Robot Global Data.vi" "Auto Left Drive"(0.0 ("Auto Left Drive")) -> ()
              n190 = global write "Robot Global Data.vi" "Auto Right Drive"(0.0 ("Auto Right Drive")) -> ()
              n191 = global write "Robot Global Data.vi" "Reset Encoder?"(FALSE ("Reset Encoder?")) -> ()
              n192 = global write "Robot Global Data.vi" "Reset Gyro?"(FALSE ("Reset Gyro?")) -> ()
              n193 = Wait (ms)(milliseconds to wait=u32 700) -> ()  [unwired: 1 out]
              n194 = call <vilib>:"CTRE_Phoenix_MotorControl_Set.vi"("Output"=w212, "Control Mode"=w211, "PhoenixMotorControlDevRef"=w213) -> ()  [unwired: 7 in, 2 out]
              n195 = call <vilib>:"CTRE_Phoenix_MotorControl_Set.vi"("Output"=w212, "Control Mode"=w211, "PhoenixMotorControlDevRef"=w214) -> ()  [unwired: 7 in, 2 out]
            }
          }
          n196 = call <vilib>:"CTRE_Phoenix_MotorControl_RefNumRegistryGet.vi"("refnum name"="BeltRight") -> ("PhoenixMotorControlDevRef"=w134:T11)  [unwired: 9 in, 1 out]
          n197 = call <vilib>:"CTRE_Phoenix_MotorControl_RefNumRegistryGet.vi"("refnum name"="BeltLeft") -> ("PhoenixMotorControlDevRef"=w135:T11)  [unwired: 9 in, 1 out]
        }
      }
    }
    frame "Switch Left" {
      n198 = case shown="\"R\"" w220 {
        frame "R" {
          n199 = disable-structure shown="Enabled" {
            frame Disabled {
              n200 = flat-sequence {
                frame #0 {
                  # "Resets things"
                  n201 = global write "Robot Global Data.vi" "Auto Left Drive"(0.0 ("Auto Left Drive")) -> ()
                  n202 = global write "Robot Global Data.vi" "Auto Right Drive"(0.0 ("Auto Right Drive")) -> ()
                  n203 = global write "Robot Global Data.vi" "Reset Encoder?"(TRUE ("Reset Encoder?")) -> ()
                  n204 = global write "Robot Global Data.vi" "Reset Gyro?"(TRUE ("Reset Gyro?")) -> ()
                  n205 = Wait (ms)(milliseconds to wait=u32 100) -> ()  [unwired: 1 out]
                }
                frame #1 {
                  n206 = while {
                    stop <- w231 stop-if-true
                    n207 = global read "Robot Global Data.vi" "EncoderValues"() -> (w236:cluster{"EncoderLeft":dbl, "EncoderRight":dbl})
                    n208 = Wait (ms)(milliseconds to wait=u32 100) -> ()  [unwired: 1 out]
                    n209 = call "Feet to Encoder Value.vi"("Feet"=15.5) -> ("Encoder Value"=w234:dbl)
                    n210 = Unbundle(w236) -> ("EncoderLeft"=w235:dbl)  [unwired: 1 out]
                    n211 = Greater Or Equal?(x=w235, y=w234) -> (x >= y?=w231:bool)
                  }
                  n212 = global write "Robot Global Data.vi" "Reset Gyro?"(FALSE ("Reset Gyro?")) -> ()
                  n213 = global write "Robot Global Data.vi" "Reset Encoder?"(FALSE ("Reset Encoder?")) -> ()
                  n214 = global write "Robot Global Data.vi" "Auto Left Drive"(0.5 ("Auto Left Drive")) -> ()
                  n215 = Wait (ms)(milliseconds to wait=u32 100) -> ()  [unwired: 1 out]
                  n216 = global write "Robot Global Data.vi" "Auto Right Drive"(-0.5 ("Auto Right Drive")) -> ()
                }
                frame #2 {
                  # "Resets things"
                  n217 = global write "Robot Global Data.vi" "Auto Right Drive"(0.0 ("Auto Right Drive")) -> ()
                  n218 = global write "Robot Global Data.vi" "Auto Left Drive"(0.0 ("Auto Left Drive")) -> ()
                  n219 = global write "Robot Global Data.vi" "Reset Encoder?"(TRUE ("Reset Encoder?")) -> ()
                  n220 = global write "Robot Global Data.vi" "Reset Gyro?"(TRUE ("Reset Gyro?")) -> ()
                  n221 = Wait (ms)(milliseconds to wait=u32 100) -> ()  [unwired: 1 out]
                }
                frame #3 {
                  n222 = global write "Robot Global Data.vi" "Reset Encoder?"(TRUE ("Reset Encoder?")) -> ()
                  n223 = global write "Robot Global Data.vi" "Reset Gyro?"(TRUE ("Reset Gyro?")) -> ()
                  n224 = global write "Robot Global Data.vi" "Auto Left Drive"(0.7 ("Auto Left Drive")) -> ()
                  n225 = global write "Robot Global Data.vi" "Auto Right Drive"(0.7 ("Auto Right Drive")) -> ()
                  n226 = Wait (ms)(milliseconds to wait=u32 600) -> ()  [unwired: 1 out]
                }
                frame #4 {
                  # "Resets things"
                  n227 = global write "Robot Global Data.vi" "Auto Right Drive"(0.0 ("Auto Right Drive")) -> ()
                  n228 = global write "Robot Global Data.vi" "Auto Left Drive"(0.0 ("Auto Left Drive")) -> ()
                  n229 = global write "Robot Global Data.vi" "Reset Encoder?"(TRUE ("Reset Encoder?")) -> ()
                  n230 = global write "Robot Global Data.vi" "Reset Gyro?"(TRUE ("Reset Gyro?")) -> ()
                  n231 = Wait (ms)(milliseconds to wait=u32 100) -> ()  [unwired: 1 out]
                }
                frame #5 {
                  n232 = while {
                    stop <- w257 stop-if-true
                    n233 = global read "Robot Global Data.vi" "EncoderValues"() -> (w262:cluster{"EncoderLeft":dbl, "EncoderRight":dbl})
                    n234 = Wait (ms)(milliseconds to wait=u32 100) -> ()  [unwired: 1 out]
                    n235 = call "Feet to Encoder Value.vi"("Feet"=12.0) -> ("Encoder Value"=w260:dbl)
                    n236 = Unbundle(w262) -> ("EncoderLeft"=w261:dbl)  [unwired: 1 out]
                    n237 = Greater Or Equal?(x=w261, y=w260) -> (x >= y?=w257:bool)
                  }
                  n238 = global write "Robot Global Data.vi" "Reset Gyro?"(FALSE ("Reset Gyro?")) -> ()
                  n239 = global write "Robot Global Data.vi" "Reset Encoder?"(FALSE ("Reset Encoder?")) -> ()
                  n240 = global write "Robot Global Data.vi" "Auto Left Drive"(0.5 ("Auto Left Drive")) -> ()
                  n241 = Wait (ms)(milliseconds to wait=u32 100) -> ()  [unwired: 1 out]
                  n242 = global write "Robot Global Data.vi" "Auto Right Drive"(-0.5 ("Auto Right Drive")) -> ()
                }
                frame #6 {
                  # "Resets things"
                  n243 = global write "Robot Global Data.vi" "Auto Right Drive"(0.0 ("Auto Right Drive")) -> ()
                  n244 = global write "Robot Global Data.vi" "Auto Left Drive"(0.0 ("Auto Left Drive")) -> ()
                  n245 = global write "Robot Global Data.vi" "Reset Encoder?"(TRUE ("Reset Encoder?")) -> ()
                  n246 = global write "Robot Global Data.vi" "Reset Gyro?"(TRUE ("Reset Gyro?")) -> ()
                  n247 = Wait (ms)(milliseconds to wait=u32 100) -> ()  [unwired: 1 out]
                }
                frame #7 {
                  n248 = global write "Robot Global Data.vi" "Reset Encoder?"(TRUE ("Reset Encoder?")) -> ()
                  n249 = global write "Robot Global Data.vi" "Reset Gyro?"(TRUE ("Reset Gyro?")) -> ()
                  n250 = global write "Robot Global Data.vi" "Auto Left Drive"(1.0 ("Auto Left Drive")) -> ()
                  n251 = global write "Robot Global Data.vi" "Auto Right Drive"(1.0 ("Auto Right Drive")) -> ()
                  n252 = Wait (ms)(milliseconds to wait=u32 450) -> ()  [unwired: 1 out]
                }
                frame #8 {
                  # "Resets things"
                  n253 = global write "Robot Global Data.vi" "Auto Right Drive"(0.0 ("Auto Right Drive")) -> ()
                  n254 = global write "Robot Global Data.vi" "Auto Left Drive"(0.0 ("Auto Left Drive")) -> ()
                  n255 = global write "Robot Global Data.vi" "Reset Encoder?"(TRUE ("Reset Encoder?")) -> ()
                  n256 = global write "Robot Global Data.vi" "Reset Gyro?"(TRUE ("Reset Gyro?")) -> ()
                  n257 = Wait (ms)(milliseconds to wait=u32 100) -> ()  [unwired: 1 out]
                }
                frame #9 {
                  n258 = global write "Robot Global Data.vi" "Reset Gyro?"(FALSE ("Reset Gyro?")) -> ()
                  n259 = global write "Robot Global Data.vi" "Reset Encoder?"(FALSE ("Reset Encoder?")) -> ()
                  n260 = global write "Robot Global Data.vi" "Auto Left Drive"(0.5 ("Auto Left Drive")) -> ()
                  n261 = Wait (ms)(milliseconds to wait=u32 1500) -> ()  [unwired: 1 out]
                  n262 = global write "Robot Global Data.vi" "Auto Right Drive"(-0.5 ("Auto Right Drive")) -> ()
                }
                frame #10 {
                  # "Resets things"
                  n263 = global write "Robot Global Data.vi" "Auto Right Drive"(0.0 ("Auto Right Drive")) -> ()
                  n264 = global write "Robot Global Data.vi" "Auto Left Drive"(0.0 ("Auto Left Drive")) -> ()
                  n265 = global write "Robot Global Data.vi" "Reset Encoder?"(TRUE ("Reset Encoder?")) -> ()
                  n266 = global write "Robot Global Data.vi" "Reset Gyro?"(TRUE ("Reset Gyro?")) -> ()
                  n267 = Wait (ms)(milliseconds to wait=u32 100) -> ()  [unwired: 1 out]
                }
                frame #11 {
                  n268 = global write "Robot Global Data.vi" "Auto Right Drive"(0.0 ("Auto Right Drive")) -> ()
                  n269 = global write "Robot Global Data.vi" "Auto Left Drive"(0.0 ("Auto Left Drive")) -> ()
                  n270 = global write "Robot Global Data.vi" "Reset Encoder?"(TRUE ("Reset Encoder?")) -> ()
                  n271 = global write "Robot Global Data.vi" "Reset Gyro?"(TRUE ("Reset Gyro?")) -> ()
                  n272 = Wait (ms)(milliseconds to wait=u32 750) -> ()  [unwired: 1 out]
                }
              }
            }
            frame Enabled {
              n273 = flat-sequence {
                frame #0 {
                  # "Resets things"
                  n274 = global write "Robot Global Data.vi" "Auto Left Drive"(0.0 ("Auto Left Drive")) -> ()
                  n275 = global write "Robot Global Data.vi" "Auto Right Drive"(0.0 ("Auto Right Drive")) -> ()
                  n276 = global write "Robot Global Data.vi" "Reset Encoder?"(TRUE ("Reset Encoder?")) -> ()
                  n277 = global write "Robot Global Data.vi" "Reset Gyro?"(TRUE ("Reset Gyro?")) -> ()
                  n278 = Wait (ms)(milliseconds to wait=u32 100) -> ()  [unwired: 1 out]
                }
                frame #1 {
                  n279 = while {
                    stop <- w303 stop-if-true
                    n280 = global read "Robot Global Data.vi" "EncoderValues"() -> (w308:cluster{"EncoderLeft":dbl, "EncoderRight":dbl})
                    n281 = Wait (ms)(milliseconds to wait=u32 100) -> ()  [unwired: 1 out]
                    n282 = call "Feet to Encoder Value.vi"("Feet"=9.0) -> ("Encoder Value"=w306:dbl)
                    n283 = Unbundle(w308) -> ("EncoderLeft"=w307:dbl)  [unwired: 1 out]
                    n284 = Greater Or Equal?(x=w307, y=w306) -> (x >= y?=w303:bool)
                  }
                  n285 = global write "Robot Global Data.vi" "Reset Gyro?"(FALSE ("Reset Gyro?")) -> ()
                  n286 = global write "Robot Global Data.vi" "Reset Encoder?"(FALSE ("Reset Encoder?")) -> ()
                  n287 = global write "Robot Global Data.vi" "Auto Left Drive"(0.5 ("Auto Left Drive")) -> ()
                  n288 = Wait (ms)(milliseconds to wait=u32 100) -> ()  [unwired: 1 out]
                  n289 = global write "Robot Global Data.vi" "Auto Right Drive"(-0.5 ("Auto Right Drive")) -> ()
                }
                frame #2 {
                  # "Resets things"
                  n290 = global write "Robot Global Data.vi" "Auto Right Drive"(0.0 ("Auto Right Drive")) -> ()
                  n291 = global write "Robot Global Data.vi" "Auto Left Drive"(0.0 ("Auto Left Drive")) -> ()
                  n292 = global write "Robot Global Data.vi" "Reset Encoder?"(TRUE ("Reset Encoder?")) -> ()
                  n293 = global write "Robot Global Data.vi" "Reset Gyro?"(TRUE ("Reset Gyro?")) -> ()
                  n294 = Wait (ms)(milliseconds to wait=u32 100) -> ()  [unwired: 1 out]
                }
              }
            }
          }
        }
        frame "L", Default {
          n295 = flat-sequence {
            tunnel: w315 -> [w359]
            tunnel: w314 -> [w360]
            frame #0 {
              # "Resets things"
              n296 = global write "Robot Global Data.vi" "Auto Left Drive"(0.0 ("Auto Left Drive")) -> ()
              n297 = global write "Robot Global Data.vi" "Auto Right Drive"(0.0 ("Auto Right Drive")) -> ()
              n298 = global write "Robot Global Data.vi" "Reset Encoder?"(TRUE ("Reset Encoder?")) -> ()
              n299 = global write "Robot Global Data.vi" "Reset Gyro?"(TRUE ("Reset Gyro?")) -> ()
              n300 = Wait (ms)(milliseconds to wait=u32 500) -> ()  [unwired: 1 out]
            }
            frame #1 {
              # "3"
              n301 = while {
                stop <- w328 stop-if-true
                n302 = global read "Robot Global Data.vi" "EncoderValues"() -> (w333:cluster{"EncoderLeft":dbl, "EncoderRight":dbl})
                n303 = Wait (ms)(milliseconds to wait=u32 100) -> ()  [unwired: 1 out]
                n304 = Unbundle(w333) -> ("EncoderLeft"=w332:dbl)  [unwired: 1 out]
                n305 = call "Feet to Encoder Value.vi"("Feet"=10.0) -> ("Encoder Value"=w331:dbl)
                n306 = Greater Or Equal?(x=w332, y=w331) -> (x >= y?=w328:bool)
              }
              n307 = global write "Robot Global Data.vi" "Reset Encoder?"(FALSE ("Reset Encoder?")) -> ()
              n308 = global write "Robot Global Data.vi" "Reset Gyro?"(FALSE ("Reset Gyro?")) -> ()
              n309 = global write "Robot Global Data.vi" "Auto Left Drive"(0.5 ("Auto Left Drive")) -> ()
              n310 = Wait (ms)(milliseconds to wait=u32 100) -> ()  [unwired: 1 out]
              n311 = global write "Robot Global Data.vi" "Auto Right Drive"(-0.5 ("Auto Right Drive")) -> ()
            }
            frame #2 {
              n312 = global write "Robot Global Data.vi" "Auto Right Drive"(0.0 ("Auto Right Drive")) -> ()
              n313 = global write "Robot Global Data.vi" "Auto Left Drive"(0.0 ("Auto Left Drive")) -> ()
              n314 = global write "Robot Global Data.vi" "Reset Encoder?"(TRUE ("Reset Encoder?")) -> ()
              n315 = global write "Robot Global Data.vi" "Reset Gyro?"(TRUE ("Reset Gyro?")) -> ()
              n316 = Wait (ms)(milliseconds to wait=u32 500) -> ()  [unwired: 1 out]
            }
            frame #3 {
              n317 = global write "Robot Global Data.vi" "Reset Gyro?"(FALSE ("Reset Gyro?")) -> ()
              n318 = global write "Robot Global Data.vi" "Reset Encoder?"(FALSE ("Reset Encoder?")) -> ()
              n319 = global write "Robot Global Data.vi" "Auto Left Drive"(0.7 ("Auto Left Drive")) -> ()
              n320 = global write "Robot Global Data.vi" "Auto Right Drive"(0.7 ("Auto Right Drive")) -> ()
              n321 = Wait (ms)(milliseconds to wait=u32 625) -> ()  [unwired: 1 out]
            }
            frame #4 {
              n322 = global write "Robot Global Data.vi" "Auto Right Drive"(0.0 ("Auto Right Drive")) -> ()
              n323 = global write "Robot Global Data.vi" "Auto Left Drive"(0.0 ("Auto Left Drive")) -> ()
              n324 = global write "Robot Global Data.vi" "Reset Encoder?"(TRUE ("Reset Encoder?")) -> ()
              n325 = global write "Robot Global Data.vi" "Reset Gyro?"(TRUE ("Reset Gyro?")) -> ()
              n326 = Wait (ms)(milliseconds to wait=u32 500) -> ()  [unwired: 1 out]
            }
            frame #5 {
              n327 = global write "Robot Global Data.vi" "Reset Gyro?"(FALSE ("Reset Gyro?")) -> ()
              n328 = global write "Robot Global Data.vi" "Reset Encoder?"(FALSE ("Reset Encoder?")) -> ()
              n329 = global write "Robot Global Data.vi" "Auto Left Drive"(0.5 ("Auto Left Drive")) -> ()
              n330 = Wait (ms)(milliseconds to wait=u32 1000) -> ()  [unwired: 1 out]
              n331 = global write "Robot Global Data.vi" "Auto Right Drive"(-0.5 ("Auto Right Drive")) -> ()
            }
            frame #6 {
              # "Resets things"
              n332 = global write "Robot Global Data.vi" "Auto Right Drive"(0.0 ("Auto Right Drive")) -> ()
              n333 = global write "Robot Global Data.vi" "Auto Left Drive"(0.0 ("Auto Left Drive")) -> ()
              n334 = global write "Robot Global Data.vi" "Reset Encoder?"(TRUE ("Reset Encoder?")) -> ()
              n335 = global write "Robot Global Data.vi" "Reset Gyro?"(TRUE ("Reset Gyro?")) -> ()
              n336 = Wait (ms)(milliseconds to wait=u32 500) -> ()  [unwired: 1 out]
            }
            frame #7 {
              w363 = T10 0 items=["PercentOutput"=0, "Position"=1, "Velocity"=2, "Current"=3, "Follower"=5, "MotionProfile"=6, "MotionMagic"=7, "MotionMagicArc"=8, "MotionProfileArc"=10, "Disabled"=15] ("Control Mode")
              w364 = T10 0 items=["PercentOutput"=0, "Position"=1, "Velocity"=2, "Current"=3, "Follower"=5, "MotionProfile"=6, "MotionMagic"=7, "MotionMagicArc"=8, "MotionProfileArc"=10, "Disabled"=15] ("Control Mode")
              # "Resets things"
              n337 = global write "Robot Global Data.vi" "Auto Left Drive"(0.0 ("Auto Left Drive")) -> ()
              n338 = global write "Robot Global Data.vi" "Auto Right Drive"(0.0 ("Auto Right Drive")) -> ()
              n339 = global write "Robot Global Data.vi" "Reset Encoder?"(FALSE ("Reset Encoder?")) -> ()
              n340 = global write "Robot Global Data.vi" "Reset Gyro?"(FALSE ("Reset Gyro?")) -> ()
              n341 = Wait (ms)(milliseconds to wait=u32 750) -> ()  [unwired: 1 out]
              n342 = call <vilib>:"CTRE_Phoenix_MotorControl_Set.vi"("Output"=0.25, "Control Mode"=w364, "PhoenixMotorControlDevRef"=w360) -> ()  [unwired: 7 in, 2 out]
              n343 = call <vilib>:"CTRE_Phoenix_MotorControl_Set.vi"("Output"=0.25, "Control Mode"=w363, "PhoenixMotorControlDevRef"=w359) -> ()  [unwired: 7 in, 2 out]
            }
          }
          n344 = call <vilib>:"CTRE_Phoenix_MotorControl_RefNumRegistryGet.vi"("refnum name"="BeltLeft") -> ("PhoenixMotorControlDevRef"=w314:T11)  [unwired: 9 in, 1 out]
          n345 = call <vilib>:"CTRE_Phoenix_MotorControl_RefNumRegistryGet.vi"("refnum name"="BeltRight") -> ("PhoenixMotorControlDevRef"=w315:T11)  [unwired: 9 in, 1 out]
        }
      }
    }
    frame "Switch Right" {
      n346 = case shown="\"L\", Default" w370 {
        frame "R" {
          n347 = flat-sequence {
            tunnel: w372 -> [w417]
            tunnel: w371 -> [w416]
            frame #0 {
              # "Resets things"
              n348 = global write "Robot Global Data.vi" "Auto Left Drive"(0.0 ("Auto Left Drive")) -> ()
              n349 = global write "Robot Global Data.vi" "Auto Right Drive"(0.0 ("Auto Right Drive")) -> ()
              n350 = global write "Robot Global Data.vi" "Reset Encoder?"(TRUE ("Reset Encoder?")) -> ()
              n351 = global write "Robot Global Data.vi" "Reset Gyro?"(TRUE ("Reset Gyro?")) -> ()
              n352 = Wait (ms)(milliseconds to wait=u32 500) -> ()  [unwired: 1 out]
            }
            frame #1 {
              # "3"
              n353 = while {
                stop <- w385 stop-if-true
                n354 = global read "Robot Global Data.vi" "EncoderValues"() -> (w390:cluster{"EncoderLeft":dbl, "EncoderRight":dbl})
                n355 = Wait (ms)(milliseconds to wait=u32 100) -> ()  [unwired: 1 out]
                n356 = Unbundle(w390) -> ("EncoderLeft"=w389:dbl)  [unwired: 1 out]
                n357 = call "Feet to Encoder Value.vi"("Feet"=10.0) -> ("Encoder Value"=w388:dbl)
                n358 = Greater Or Equal?(x=w389, y=w388) -> (x >= y?=w385:bool)
              }
              n359 = global write "Robot Global Data.vi" "Reset Encoder?"(FALSE ("Reset Encoder?")) -> ()
              n360 = global write "Robot Global Data.vi" "Reset Gyro?"(FALSE ("Reset Gyro?")) -> ()
              n361 = global write "Robot Global Data.vi" "Auto Left Drive"(0.5 ("Auto Left Drive")) -> ()
              n362 = Wait (ms)(milliseconds to wait=u32 100) -> ()  [unwired: 1 out]
              n363 = global write "Robot Global Data.vi" "Auto Right Drive"(-0.5 ("Auto Right Drive")) -> ()
            }
            frame #2 {
              n364 = global write "Robot Global Data.vi" "Auto Right Drive"(0.0 ("Auto Right Drive")) -> ()
              n365 = global write "Robot Global Data.vi" "Auto Left Drive"(0.0 ("Auto Left Drive")) -> ()
              n366 = global write "Robot Global Data.vi" "Reset Encoder?"(TRUE ("Reset Encoder?")) -> ()
              n367 = global write "Robot Global Data.vi" "Reset Gyro?"(TRUE ("Reset Gyro?")) -> ()
              n368 = Wait (ms)(milliseconds to wait=u32 500) -> ()  [unwired: 1 out]
            }
            frame #3 {
              n369 = global write "Robot Global Data.vi" "Reset Gyro?"(FALSE ("Reset Gyro?")) -> ()
              n370 = global write "Robot Global Data.vi" "Reset Encoder?"(FALSE ("Reset Encoder?")) -> ()
              n371 = global write "Robot Global Data.vi" "Auto Left Drive"(0.7 ("Auto Left Drive")) -> ()
              n372 = global write "Robot Global Data.vi" "Auto Right Drive"(0.7 ("Auto Right Drive")) -> ()
              n373 = Wait (ms)(milliseconds to wait=u32 625) -> ()  [unwired: 1 out]
            }
            frame #4 {
              n374 = global write "Robot Global Data.vi" "Auto Right Drive"(0.0 ("Auto Right Drive")) -> ()
              n375 = global write "Robot Global Data.vi" "Auto Left Drive"(0.0 ("Auto Left Drive")) -> ()
              n376 = global write "Robot Global Data.vi" "Reset Encoder?"(TRUE ("Reset Encoder?")) -> ()
              n377 = global write "Robot Global Data.vi" "Reset Gyro?"(TRUE ("Reset Gyro?")) -> ()
              n378 = Wait (ms)(milliseconds to wait=u32 500) -> ()  [unwired: 1 out]
            }
            frame #5 {
              n379 = global write "Robot Global Data.vi" "Reset Gyro?"(FALSE ("Reset Gyro?")) -> ()
              n380 = global write "Robot Global Data.vi" "Reset Encoder?"(FALSE ("Reset Encoder?")) -> ()
              n381 = global write "Robot Global Data.vi" "Auto Left Drive"(0.5 ("Auto Left Drive")) -> ()
              n382 = Wait (ms)(milliseconds to wait=u32 1000) -> ()  [unwired: 1 out]
              n383 = global write "Robot Global Data.vi" "Auto Right Drive"(-0.5 ("Auto Right Drive")) -> ()
            }
            frame #6 {
              # "Resets things"
              n384 = global write "Robot Global Data.vi" "Auto Right Drive"(0.0 ("Auto Right Drive")) -> ()
              n385 = global write "Robot Global Data.vi" "Auto Left Drive"(0.0 ("Auto Left Drive")) -> ()
              n386 = global write "Robot Global Data.vi" "Reset Encoder?"(TRUE ("Reset Encoder?")) -> ()
              n387 = global write "Robot Global Data.vi" "Reset Gyro?"(TRUE ("Reset Gyro?")) -> ()
              n388 = Wait (ms)(milliseconds to wait=u32 500) -> ()  [unwired: 1 out]
            }
            frame #7 {
              w420 = T10 0 items=["PercentOutput"=0, "Position"=1, "Velocity"=2, "Current"=3, "Follower"=5, "MotionProfile"=6, "MotionMagic"=7, "MotionMagicArc"=8, "MotionProfileArc"=10, "Disabled"=15] ("Control Mode")
              w421 = T10 0 items=["PercentOutput"=0, "Position"=1, "Velocity"=2, "Current"=3, "Follower"=5, "MotionProfile"=6, "MotionMagic"=7, "MotionMagicArc"=8, "MotionProfileArc"=10, "Disabled"=15] ("Control Mode")
              # "Resets things"
              n389 = global write "Robot Global Data.vi" "Auto Left Drive"(0.0 ("Auto Left Drive")) -> ()
              n390 = global write "Robot Global Data.vi" "Auto Right Drive"(0.0 ("Auto Right Drive")) -> ()
              n391 = global write "Robot Global Data.vi" "Reset Encoder?"(FALSE ("Reset Encoder?")) -> ()
              n392 = global write "Robot Global Data.vi" "Reset Gyro?"(FALSE ("Reset Gyro?")) -> ()
              n393 = Wait (ms)(milliseconds to wait=u32 750) -> ()  [unwired: 1 out]
              n394 = call <vilib>:"CTRE_Phoenix_MotorControl_Set.vi"("Output"=0.25, "Control Mode"=w421, "PhoenixMotorControlDevRef"=w417) -> ()  [unwired: 7 in, 2 out]
              n395 = call <vilib>:"CTRE_Phoenix_MotorControl_Set.vi"("Output"=0.25, "Control Mode"=w420, "PhoenixMotorControlDevRef"=w416) -> ()  [unwired: 7 in, 2 out]
            }
          }
          n396 = call <vilib>:"CTRE_Phoenix_MotorControl_RefNumRegistryGet.vi"("refnum name"="BeltLeft") -> ("PhoenixMotorControlDevRef"=w372:T11)  [unwired: 9 in, 1 out]
          n397 = call <vilib>:"CTRE_Phoenix_MotorControl_RefNumRegistryGet.vi"("refnum name"="BeltRight") -> ("PhoenixMotorControlDevRef"=w371:T11)  [unwired: 9 in, 1 out]
        }
        frame "L", Default {
          n398 = disable-structure shown="Enabled" {
            frame Disabled {
              n399 = flat-sequence {
                frame #0 {
                  # "Resets things"
                  n400 = global write "Robot Global Data.vi" "Auto Left Drive"(0.0 ("Auto Left Drive")) -> ()
                  n401 = global write "Robot Global Data.vi" "Auto Right Drive"(0.0 ("Auto Right Drive")) -> ()
                  n402 = global write "Robot Global Data.vi" "Reset Encoder?"(TRUE ("Reset Encoder?")) -> ()
                  n403 = global write "Robot Global Data.vi" "Reset Gyro?"(TRUE ("Reset Gyro?")) -> ()
                  n404 = Wait (ms)(milliseconds to wait=u32 100) -> ()  [unwired: 1 out]
                }
                frame #1 {
                  n405 = while {
                    stop <- w437 stop-if-true
                    n406 = global read "Robot Global Data.vi" "EncoderValues"() -> (w442:cluster{"EncoderLeft":dbl, "EncoderRight":dbl})
                    n407 = Wait (ms)(milliseconds to wait=u32 100) -> ()  [unwired: 1 out]
                    n408 = call "Feet to Encoder Value.vi"("Feet"=15.5) -> ("Encoder Value"=w440:dbl)
                    n409 = Unbundle(w442) -> ("EncoderLeft"=w441:dbl)  [unwired: 1 out]
                    n410 = Greater Or Equal?(x=w441, y=w440) -> (x >= y?=w437:bool)
                  }
                  n411 = global write "Robot Global Data.vi" "Reset Gyro?"(FALSE ("Reset Gyro?")) -> ()
                  n412 = global write "Robot Global Data.vi" "Reset Encoder?"(FALSE ("Reset Encoder?")) -> ()
                  n413 = global write "Robot Global Data.vi" "Auto Left Drive"(0.5 ("Auto Left Drive")) -> ()
                  n414 = Wait (ms)(milliseconds to wait=u32 100) -> ()  [unwired: 1 out]
                  n415 = global write "Robot Global Data.vi" "Auto Right Drive"(-0.5 ("Auto Right Drive")) -> ()
                }
                frame #2 {
                  # "Resets things"
                  n416 = global write "Robot Global Data.vi" "Auto Right Drive"(0.0 ("Auto Right Drive")) -> ()
                  n417 = global write "Robot Global Data.vi" "Auto Left Drive"(0.0 ("Auto Left Drive")) -> ()
                  n418 = global write "Robot Global Data.vi" "Reset Encoder?"(TRUE ("Reset Encoder?")) -> ()
                  n419 = global write "Robot Global Data.vi" "Reset Gyro?"(TRUE ("Reset Gyro?")) -> ()
                  n420 = Wait (ms)(milliseconds to wait=u32 100) -> ()  [unwired: 1 out]
                }
                frame #3 {
                  n421 = global write "Robot Global Data.vi" "Reset Encoder?"(TRUE ("Reset Encoder?")) -> ()
                  n422 = global write "Robot Global Data.vi" "Reset Gyro?"(TRUE ("Reset Gyro?")) -> ()
                  n423 = global write "Robot Global Data.vi" "Auto Left Drive"(-0.7 ("Auto Left Drive")) -> ()
                  n424 = global write "Robot Global Data.vi" "Auto Right Drive"(-0.7 ("Auto Right Drive")) -> ()
                  n425 = Wait (ms)(milliseconds to wait=u32 600) -> ()  [unwired: 1 out]
                }
                frame #4 {
                  # "Resets things"
                  n426 = global write "Robot Global Data.vi" "Auto Right Drive"(0.0 ("Auto Right Drive")) -> ()
                  n427 = global write "Robot Global Data.vi" "Auto Left Drive"(0.0 ("Auto Left Drive")) -> ()
                  n428 = global write "Robot Global Data.vi" "Reset Encoder?"(TRUE ("Reset Encoder?")) -> ()
                  n429 = global write "Robot Global Data.vi" "Reset Gyro?"(TRUE ("Reset Gyro?")) -> ()
                  n430 = Wait (ms)(milliseconds to wait=u32 100) -> ()  [unwired: 1 out]
                }
                frame #5 {
                  n431 = while {
                    stop <- w463 stop-if-true
                    n432 = global read "Robot Global Data.vi" "EncoderValues"() -> (w468:cluster{"EncoderLeft":dbl, "EncoderRight":dbl})
                    n433 = Wait (ms)(milliseconds to wait=u32 100) -> ()  [unwired: 1 out]
                    n434 = call "Feet to Encoder Value.vi"("Feet"=12.0) -> ("Encoder Value"=w466:dbl)
                    n435 = Unbundle(w468) -> ("EncoderLeft"=w467:dbl)  [unwired: 1 out]
                    n436 = Greater Or Equal?(x=w467, y=w466) -> (x >= y?=w463:bool)
                  }
                  n437 = global write "Robot Global Data.vi" "Reset Gyro?"(FALSE ("Reset Gyro?")) -> ()
                  n438 = global write "Robot Global Data.vi" "Reset Encoder?"(FALSE ("Reset Encoder?")) -> ()
                  n439 = global write "Robot Global Data.vi" "Auto Left Drive"(0.5 ("Auto Left Drive")) -> ()
                  n440 = Wait (ms)(milliseconds to wait=u32 100) -> ()  [unwired: 1 out]
                  n441 = global write "Robot Global Data.vi" "Auto Right Drive"(-0.5 ("Auto Right Drive")) -> ()
                }
                frame #6 {
                  # "Resets things"
                  n442 = global write "Robot Global Data.vi" "Auto Right Drive"(0.0 ("Auto Right Drive")) -> ()
                  n443 = global write "Robot Global Data.vi" "Auto Left Drive"(0.0 ("Auto Left Drive")) -> ()
                  n444 = global write "Robot Global Data.vi" "Reset Encoder?"(TRUE ("Reset Encoder?")) -> ()
                  n445 = global write "Robot Global Data.vi" "Reset Gyro?"(TRUE ("Reset Gyro?")) -> ()
                  n446 = Wait (ms)(milliseconds to wait=u32 100) -> ()  [unwired: 1 out]
                }
                frame #7 {
                  n447 = global write "Robot Global Data.vi" "Reset Encoder?"(TRUE ("Reset Encoder?")) -> ()
                  n448 = global write "Robot Global Data.vi" "Reset Gyro?"(TRUE ("Reset Gyro?")) -> ()
                  n449 = global write "Robot Global Data.vi" "Auto Left Drive"(-1.0 ("Auto Left Drive")) -> ()
                  n450 = global write "Robot Global Data.vi" "Auto Right Drive"(-1.0 ("Auto Right Drive")) -> ()
                  n451 = Wait (ms)(milliseconds to wait=u32 450) -> ()  [unwired: 1 out]
                }
                frame #8 {
                  # "Resets things"
                  n452 = global write "Robot Global Data.vi" "Auto Right Drive"(0.0 ("Auto Right Drive")) -> ()
                  n453 = global write "Robot Global Data.vi" "Auto Left Drive"(0.0 ("Auto Left Drive")) -> ()
                  n454 = global write "Robot Global Data.vi" "Reset Encoder?"(TRUE ("Reset Encoder?")) -> ()
                  n455 = global write "Robot Global Data.vi" "Reset Gyro?"(TRUE ("Reset Gyro?")) -> ()
                  n456 = Wait (ms)(milliseconds to wait=u32 100) -> ()  [unwired: 1 out]
                }
                frame #9 {
                  n457 = global write "Robot Global Data.vi" "Reset Gyro?"(FALSE ("Reset Gyro?")) -> ()
                  n458 = global write "Robot Global Data.vi" "Reset Encoder?"(FALSE ("Reset Encoder?")) -> ()
                  n459 = global write "Robot Global Data.vi" "Auto Left Drive"(0.5 ("Auto Left Drive")) -> ()
                  n460 = Wait (ms)(milliseconds to wait=u32 1500) -> ()  [unwired: 1 out]
                  n461 = global write "Robot Global Data.vi" "Auto Right Drive"(-0.5 ("Auto Right Drive")) -> ()
                }
                frame #10 {
                  # "Resets things"
                  n462 = global write "Robot Global Data.vi" "Auto Right Drive"(0.0 ("Auto Right Drive")) -> ()
                  n463 = global write "Robot Global Data.vi" "Auto Left Drive"(0.0 ("Auto Left Drive")) -> ()
                  n464 = global write "Robot Global Data.vi" "Reset Encoder?"(TRUE ("Reset Encoder?")) -> ()
                  n465 = global write "Robot Global Data.vi" "Reset Gyro?"(TRUE ("Reset Gyro?")) -> ()
                  n466 = Wait (ms)(milliseconds to wait=u32 100) -> ()  [unwired: 1 out]
                }
                frame #11 {
                  n467 = global write "Robot Global Data.vi" "Auto Right Drive"(0.0 ("Auto Right Drive")) -> ()
                  n468 = global write "Robot Global Data.vi" "Auto Left Drive"(0.0 ("Auto Left Drive")) -> ()
                  n469 = global write "Robot Global Data.vi" "Reset Encoder?"(TRUE ("Reset Encoder?")) -> ()
                  n470 = global write "Robot Global Data.vi" "Reset Gyro?"(TRUE ("Reset Gyro?")) -> ()
                  n471 = Wait (ms)(milliseconds to wait=u32 750) -> ()  [unwired: 1 out]
                }
              }
            }
            frame Enabled {
              n472 = flat-sequence {
                frame #0 {
                  # "Resets things"
                  n473 = global write "Robot Global Data.vi" "Auto Left Drive"(0.0 ("Auto Left Drive")) -> ()
                  n474 = global write "Robot Global Data.vi" "Auto Right Drive"(0.0 ("Auto Right Drive")) -> ()
                  n475 = global write "Robot Global Data.vi" "Reset Encoder?"(TRUE ("Reset Encoder?")) -> ()
                  n476 = global write "Robot Global Data.vi" "Reset Gyro?"(TRUE ("Reset Gyro?")) -> ()
                  n477 = Wait (ms)(milliseconds to wait=u32 100) -> ()  [unwired: 1 out]
                }
                frame #1 {
                  n478 = while {
                    stop <- w509 stop-if-true
                    n479 = global read "Robot Global Data.vi" "EncoderValues"() -> (w514:cluster{"EncoderLeft":dbl, "EncoderRight":dbl})
                    n480 = Wait (ms)(milliseconds to wait=u32 100) -> ()  [unwired: 1 out]
                    n481 = call "Feet to Encoder Value.vi"("Feet"=9.0) -> ("Encoder Value"=w512:dbl)
                    n482 = Unbundle(w514) -> ("EncoderLeft"=w513:dbl)  [unwired: 1 out]
                    n483 = Greater Or Equal?(x=w513, y=w512) -> (x >= y?=w509:bool)
                  }
                  n484 = global write "Robot Global Data.vi" "Reset Gyro?"(FALSE ("Reset Gyro?")) -> ()
                  n485 = global write "Robot Global Data.vi" "Reset Encoder?"(FALSE ("Reset Encoder?")) -> ()
                  n486 = global write "Robot Global Data.vi" "Auto Left Drive"(0.5 ("Auto Left Drive")) -> ()
                  n487 = Wait (ms)(milliseconds to wait=u32 100) -> ()  [unwired: 1 out]
                  n488 = global write "Robot Global Data.vi" "Auto Right Drive"(-0.5 ("Auto Right Drive")) -> ()
                }
                frame #2 {
                  # "Resets things"
                  n489 = global write "Robot Global Data.vi" "Auto Right Drive"(0.0 ("Auto Right Drive")) -> ()
                  n490 = global write "Robot Global Data.vi" "Auto Left Drive"(0.0 ("Auto Left Drive")) -> ()
                  n491 = global write "Robot Global Data.vi" "Reset Encoder?"(TRUE ("Reset Encoder?")) -> ()
                  n492 = global write "Robot Global Data.vi" "Reset Gyro?"(TRUE ("Reset Gyro?")) -> ()
                  n493 = Wait (ms)(milliseconds to wait=u32 100) -> ()  [unwired: 1 out]
                }
              }
            }
          }
        }
      }
    }
    frame "Scale Left" {
      (unwired) "BeltLeft" ("refnum name")
      n494 = flat-sequence {
        tunnel: w520 -> [w546]
        tunnel: w527 -> [w566]
        tunnel: w526 -> [w565]
        tunnel: w524 -> [w564]
        tunnel: w522 -> [w579]
        tunnel: w521 -> [w578]
        frame #0 {
          # "Resets things"
          n495 = global write "Robot Global Data.vi" "Auto Right Drive"(0.0 ("Auto Right Drive")) -> ()
          n496 = global write "Robot Global Data.vi" "Reset Gyro?"(TRUE ("Reset Gyro?")) -> ()
          n497 = global write "Robot Global Data.vi" "Auto Left Drive"(0.0 ("Auto Left Drive")) -> ()
          n498 = global write "Robot Global Data.vi" "Reset Encoder?"(TRUE ("Reset Encoder?")) -> ()
          n499 = Wait (ms)(milliseconds to wait=u32 100) -> ()  [unwired: 1 out]
        }
        frame #1 {
          n500 = while {
            stop <- w540 stop-if-true
            n501 = global read "Robot Global Data.vi" "EncoderValues"() -> (w545:cluster{"EncoderLeft":dbl, "EncoderRight":dbl})
            n502 = Wait (ms)(milliseconds to wait=u32 100) -> ()  [unwired: 1 out]
            n503 = call "Feet to Encoder Value.vi"("Feet"=17.0) -> ("Encoder Value"=w543:dbl)
            n504 = Unbundle(w545) -> ("EncoderLeft"=w544:dbl)  [unwired: 1 out]
            n505 = Greater Or Equal?(x=w544, y=w543) -> (x >= y?=w540:bool)
          }
          n506 = global write "Robot Global Data.vi" "Reset Gyro?"(FALSE ("Reset Gyro?")) -> ()
          n507 = global write "Robot Global Data.vi" "Reset Encoder?"(FALSE ("Reset Encoder?")) -> ()
          n508 = global write "Robot Global Data.vi" "Auto Left Drive"(0.5 ("Auto Left Drive")) -> ()
          n509 = Wait (ms)(milliseconds to wait=u32 100) -> ()  [unwired: 1 out]
          n510 = global write "Robot Global Data.vi" "Auto Right Drive"(-0.5 ("Auto Right Drive")) -> ()
        }
        frame #2 {
          # "Resets things"
          n511 = while {
            tunnel: w546 -> [w552]
            stop <- w554 stop-if-true
            n512 = Wait (ms)(milliseconds to wait=u32 100) -> ()  [unwired: 1 out]
            n513 = Less Or Equal?(x=w552, y=90.0) -> (x <= y?=w554:bool)
          }
          n514 = Wait (ms)(milliseconds to wait=u32 250) -> ()  [unwired: 1 out]
          n515 = global write "Robot Global Data.vi" "Auto Right Drive"(0.7 ("Auto Right Drive")) -> ()
          n516 = global write "Robot Global Data.vi" "Auto Left Drive"(0.7 ("Auto Left Drive")) -> ()
          n517 = global write "Robot Global Data.vi" "Reset Encoder?"(TRUE ("Reset Encoder?")) -> ()
          n518 = global write "Robot Global Data.vi" "Reset Gyro?"(TRUE ("Reset Gyro?")) -> ()
        }
        frame #3 {
          w557 = -0.9 ("Output")
          w559 = T10 0 items=["PercentOutput"=0, "Position"=1, "Velocity"=2, "Current"=3, "Follower"=5, "MotionProfile"=6, "MotionMagic"=7, "MotionMagicArc"=8, "MotionProfileArc"=10, "Disabled"=15] ("Control Mode")
          n519 = call <vilib>:"CTRE_Phoenix_MotorControl_Set.vi"("Output"=1.0, "Control Mode"=w559, "PhoenixMotorControlDevRef"=w564) -> ()  [unwired: 7 in, 2 out]
          n520 = call <vilib>:"CTRE_Phoenix_MotorControl_Set.vi"("Output"=w557, "Control Mode"=w559, "PhoenixMotorControlDevRef"=w565) -> ()  [unwired: 7 in, 2 out]
          n521 = call <vilib>:"CTRE_Phoenix_MotorControl_Set.vi"("Output"=w557, "Control Mode"=w559, "PhoenixMotorControlDevRef"=w566) -> ()  [unwired: 7 in, 2 out]
          n522 = global write "Robot Global Data.vi" "Reset Gyro?"(TRUE ("Reset Gyro?")) -> ()
          n523 = Wait (ms)(milliseconds to wait=u32 400) -> ()  [unwired: 1 out]
          n524 = global write "Robot Global Data.vi" "Auto Right Drive"(0.0 ("Auto Right Drive")) -> ()
          n525 = global write "Robot Global Data.vi" "Auto Left Drive"(0.0 ("Auto Left Drive")) -> ()
          n526 = global write "Robot Global Data.vi" "Reset Encoder?"(TRUE ("Reset Encoder?")) -> ()
        }
        frame #4 {
          # "Resets things"
          n527 = global write "Robot Global Data.vi" "Auto Right Drive"(0.0 ("Auto Right Drive")) -> ()
          n528 = global write "Robot Global Data.vi" "Auto Left Drive"(0.0 ("Auto Left Drive")) -> ()
          n529 = global write "Robot Global Data.vi" "Reset Gyro?"(TRUE ("Reset Gyro?")) -> ()
          n530 = global write "Robot Global Data.vi" "Reset Encoder?"(TRUE ("Reset Encoder?")) -> ()
          n531 = Wait (ms)(milliseconds to wait=u32 100) -> ()  [unwired: 1 out]
        }
        frame #5 {
          w577 = 0.4 ("Output")
          w580 = T10 0 items=["PercentOutput"=0, "Position"=1, "Velocity"=2, "Current"=3, "Follower"=5, "MotionProfile"=6, "MotionMagic"=7, "MotionMagicArc"=8, "MotionProfileArc"=10, "Disabled"=15] ("Control Mode")
          # "Resets things"
          n532 = global write "Robot Global Data.vi" "Auto Left Drive"(0.0 ("Auto Left Drive")) -> ()
          n533 = global write "Robot Global Data.vi" "Reset Gyro?"(TRUE ("Reset Gyro?")) -> ()
          n534 = global write "Robot Global Data.vi" "Auto Right Drive"(0.0 ("Auto Right Drive")) -> ()
          n535 = global write "Robot Global Data.vi" "Reset Encoder?"(TRUE ("Reset Encoder?")) -> ()
          n536 = Wait (ms)(milliseconds to wait=u32 1000) -> ()  [unwired: 1 out]
          n537 = call <vilib>:"CTRE_Phoenix_MotorControl_Set.vi"("Output"=w577, "Control Mode"=w580, "PhoenixMotorControlDevRef"=w579) -> ()  [unwired: 7 in, 2 out]
          n538 = call <vilib>:"CTRE_Phoenix_MotorControl_Set.vi"("Output"=w577, "Control Mode"=w580, "PhoenixMotorControlDevRef"=w578) -> ()  [unwired: 7 in, 2 out]
        }
      }
      n539 = call <vilib>:"CTRE_Phoenix_MotorControl_RefNumRegistryGet.vi"("refnum name"="Arm") -> ("PhoenixMotorControlDevRef"=w524:T11)  [unwired: 9 in, 1 out]
      n540 = call <vilib>:"CTRE_Phoenix_MotorControl_RefNumRegistryGet.vi"("refnum name"="Elbow 2") -> ("PhoenixMotorControlDevRef"=w526:T11)  [unwired: 9 in, 1 out]
      n541 = call <vilib>:"CTRE_Phoenix_MotorControl_RefNumRegistryGet.vi"("refnum name"="Elbow") -> ("PhoenixMotorControlDevRef"=w527:T11)  [unwired: 9 in, 1 out]
      n542 = call <vilib>:"CTRE_Phoenix_MotorControl_RefNumRegistryGet.vi"() -> ("PhoenixMotorControlDevRef"=w522:T11)  [unwired: 10 in, 1 out]
      n543 = call <vilib>:"CTRE_Phoenix_MotorControl_RefNumRegistryGet.vi"("refnum name"="BeltRight") -> ("PhoenixMotorControlDevRef"=w521:T11)  [unwired: 9 in, 1 out]
    }
    frame "Scale Right" {
    }
    frame "Line Right" {
      n544 = case shown="\"L\"" w581 {
        frame "L" {
          n545 = flat-sequence {
            frame #0 {
              # "Resets things"
              n546 = global write "Robot Global Data.vi" "Auto Left Drive"(0.0 ("Auto Left Drive")) -> ()
              n547 = global write "Robot Global Data.vi" "Auto Right Drive"(0.0 ("Auto Right Drive")) -> ()
              n548 = global write "Robot Global Data.vi" "Reset Encoder?"(TRUE ("Reset Encoder?")) -> ()
              n549 = global write "Robot Global Data.vi" "Reset Gyro?"(TRUE ("Reset Gyro?")) -> ()
              n550 = Wait (ms)(milliseconds to wait=u32 100) -> ()  [unwired: 1 out]
            }
            frame #1 {
              n551 = while {
                stop <- w592 stop-if-true
                n552 = global read "Robot Global Data.vi" "EncoderValues"() -> (w597:cluster{"EncoderLeft":dbl, "EncoderRight":dbl})
                n553 = Wait (ms)(milliseconds to wait=u32 100) -> ()  [unwired: 1 out]
                n554 = call "Feet to Encoder Value.vi"("Feet"=12.0) -> ("Encoder Value"=w595:dbl)
                n555 = Unbundle(w597) -> ("EncoderLeft"=w596:dbl)  [unwired: 1 out]
                n556 = Greater Or Equal?(x=w596, y=w595) -> (x >= y?=w592:bool)
              }
              n557 = global write "Robot Global Data.vi" "Reset Gyro?"(FALSE ("Reset Gyro?")) -> ()
              n558 = global write "Robot Global Data.vi" "Reset Encoder?"(FALSE ("Reset Encoder?")) -> ()
              n559 = global write "Robot Global Data.vi" "Auto Left Drive"(0.5 ("Auto Left Drive")) -> ()
              n560 = Wait (ms)(milliseconds to wait=u32 100) -> ()  [unwired: 1 out]
              n561 = global write "Robot Global Data.vi" "Auto Right Drive"(-0.5 ("Auto Right Drive")) -> ()
            }
            frame #2 {
              # "Resets things"
              n562 = global write "Robot Global Data.vi" "Auto Right Drive"(0.0 ("Auto Right Drive")) -> ()
              n563 = global write "Robot Global Data.vi" "Auto Left Drive"(0.0 ("Auto Left Drive")) -> ()
              n564 = global write "Robot Global Data.vi" "Reset Encoder?"(TRUE ("Reset Encoder?")) -> ()
              n565 = global write "Robot Global Data.vi" "Reset Gyro?"(TRUE ("Reset Gyro?")) -> ()
              n566 = Wait (ms)(milliseconds to wait=u32 100) -> ()  [unwired: 1 out]
            }
            frame #3 {
              n567 = global write "Robot Global Data.vi" "Reset Encoder?"(TRUE ("Reset Encoder?")) -> ()
              n568 = global write "Robot Global Data.vi" "Reset Gyro?"(TRUE ("Reset Gyro?")) -> ()
              n569 = global write "Robot Global Data.vi" "Auto Left Drive"(-0.7 ("Auto Left Drive")) -> ()
              n570 = global write "Robot Global Data.vi" "Auto Right Drive"(-0.7 ("Auto Right Drive")) -> ()
              n571 = Wait (ms)(milliseconds to wait=u32 650) -> ()  [unwired: 1 out]
            }
            frame #4 {
              # "Resets things"
              n572 = global write "Robot Global Data.vi" "Auto Right Drive"(0.0 ("Auto Right Drive")) -> ()
              n573 = global write "Robot Global Data.vi" "Auto Left Drive"(0.0 ("Auto Left Drive")) -> ()
              n574 = global write "Robot Global Data.vi" "Reset Encoder?"(TRUE ("Reset Encoder?")) -> ()
              n575 = global write "Robot Global Data.vi" "Reset Gyro?"(TRUE ("Reset Gyro?")) -> ()
              n576 = Wait (ms)(milliseconds to wait=u32 100) -> ()  [unwired: 1 out]
            }
            frame #5 {
              n577 = while {
                stop <- w618 stop-if-true
                n578 = global read "Robot Global Data.vi" "EncoderValues"() -> (w623:cluster{"EncoderLeft":dbl, "EncoderRight":dbl})
                n579 = Wait (ms)(milliseconds to wait=u32 100) -> ()  [unwired: 1 out]
                n580 = call "Feet to Encoder Value.vi"("Feet"=14.0) -> ("Encoder Value"=w621:dbl)
                n581 = Unbundle(w623) -> ("EncoderLeft"=w622:dbl)  [unwired: 1 out]
                n582 = Greater Or Equal?(x=w622, y=w621) -> (x >= y?=w618:bool)
              }
              n583 = global write "Robot Global Data.vi" "Reset Gyro?"(FALSE ("Reset Gyro?")) -> ()
              n584 = global write "Robot Global Data.vi" "Reset Encoder?"(FALSE ("Reset Encoder?")) -> ()
              n585 = global write "Robot Global Data.vi" "Auto Left Drive"(0.5 ("Auto Left Drive")) -> ()
              n586 = Wait (ms)(milliseconds to wait=u32 100) -> ()  [unwired: 1 out]
              n587 = global write "Robot Global Data.vi" "Auto Right Drive"(-0.5 ("Auto Right Drive")) -> ()
            }
            frame #6 {
              # "Resets things"
              n588 = global write "Robot Global Data.vi" "Auto Right Drive"(0.0 ("Auto Right Drive")) -> ()
              n589 = global write "Robot Global Data.vi" "Auto Left Drive"(0.0 ("Auto Left Drive")) -> ()
              n590 = global write "Robot Global Data.vi" "Reset Encoder?"(TRUE ("Reset Encoder?")) -> ()
              n591 = global write "Robot Global Data.vi" "Reset Gyro?"(TRUE ("Reset Gyro?")) -> ()
              n592 = Wait (ms)(milliseconds to wait=u32 100) -> ()  [unwired: 1 out]
            }
            frame #7 {
              n593 = global write "Robot Global Data.vi" "Reset Encoder?"(TRUE ("Reset Encoder?")) -> ()
              n594 = global write "Robot Global Data.vi" "Reset Gyro?"(TRUE ("Reset Gyro?")) -> ()
              n595 = global write "Robot Global Data.vi" "Auto Left Drive"(-0.7 ("Auto Left Drive")) -> ()
              n596 = global write "Robot Global Data.vi" "Auto Right Drive"(-0.7 ("Auto Right Drive")) -> ()
              n597 = Wait (ms)(milliseconds to wait=u32 650) -> ()  [unwired: 1 out]
            }
            frame #8 {
              # "Resets things"
              n598 = global write "Robot Global Data.vi" "Auto Right Drive"(0.0 ("Auto Right Drive")) -> ()
              n599 = global write "Robot Global Data.vi" "Auto Left Drive"(0.0 ("Auto Left Drive")) -> ()
              n600 = global write "Robot Global Data.vi" "Reset Encoder?"(TRUE ("Reset Encoder?")) -> ()
              n601 = global write "Robot Global Data.vi" "Reset Gyro?"(TRUE ("Reset Gyro?")) -> ()
              n602 = Wait (ms)(milliseconds to wait=u32 100) -> ()  [unwired: 1 out]
            }
            frame #9 {
              n603 = global write "Robot Global Data.vi" "Reset Gyro?"(FALSE ("Reset Gyro?")) -> ()
              n604 = global write "Robot Global Data.vi" "Reset Encoder?"(FALSE ("Reset Encoder?")) -> ()
              n605 = global write "Robot Global Data.vi" "Auto Left Drive"(0.5 ("Auto Left Drive")) -> ()
              n606 = Wait (ms)(milliseconds to wait=u32 1500) -> ()  [unwired: 1 out]
              n607 = global write "Robot Global Data.vi" "Auto Right Drive"(-0.5 ("Auto Right Drive")) -> ()
            }
            frame #10 {
              # "Resets things"
              n608 = global write "Robot Global Data.vi" "Auto Right Drive"(0.0 ("Auto Right Drive")) -> ()
              n609 = global write "Robot Global Data.vi" "Auto Left Drive"(0.0 ("Auto Left Drive")) -> ()
              n610 = global write "Robot Global Data.vi" "Reset Encoder?"(TRUE ("Reset Encoder?")) -> ()
              n611 = global write "Robot Global Data.vi" "Reset Gyro?"(TRUE ("Reset Gyro?")) -> ()
              n612 = Wait (ms)(milliseconds to wait=u32 100) -> ()  [unwired: 1 out]
            }
            frame #11 {
              n613 = global write "Robot Global Data.vi" "Auto Right Drive"(0.0 ("Auto Right Drive")) -> ()
              n614 = global write "Robot Global Data.vi" "Auto Left Drive"(0.0 ("Auto Left Drive")) -> ()
              n615 = global write "Robot Global Data.vi" "Reset Encoder?"(TRUE ("Reset Encoder?")) -> ()
              n616 = global write "Robot Global Data.vi" "Reset Gyro?"(TRUE ("Reset Gyro?")) -> ()
              n617 = Wait (ms)(milliseconds to wait=u32 750) -> ()  [unwired: 1 out]
            }
          }
        }
        frame "R", Default {
          n618 = flat-sequence {
            frame #0 {
              # "Resets things"
              n619 = global write "Robot Global Data.vi" "Auto Left Drive"(0.0 ("Auto Left Drive")) -> ()
              n620 = global write "Robot Global Data.vi" "Auto Right Drive"(0.0 ("Auto Right Drive")) -> ()
              n621 = global write "Robot Global Data.vi" "Reset Encoder?"(TRUE ("Reset Encoder?")) -> ()
              n622 = global write "Robot Global Data.vi" "Reset Gyro?"(TRUE ("Reset Gyro?")) -> ()
              n623 = Wait (ms)(milliseconds to wait=u32 100) -> ()  [unwired: 1 out]
            }
            frame #1 {
              n624 = while {
                stop <- w664 stop-if-true
                n625 = global read "Robot Global Data.vi" "EncoderValues"() -> (w669:cluster{"EncoderLeft":dbl, "EncoderRight":dbl})
                n626 = Wait (ms)(milliseconds to wait=u32 100) -> ()  [unwired: 1 out]
                n627 = call "Feet to Encoder Value.vi"("Feet"=9.0) -> ("Encoder Value"=w667:dbl)
                n628 = Unbundle(w669) -> ("EncoderLeft"=w668:dbl)  [unwired: 1 out]
                n629 = Greater Or Equal?(x=w668, y=w667) -> (x >= y?=w664:bool)
              }
              n630 = global write "Robot Global Data.vi" "Reset Gyro?"(FALSE ("Reset Gyro?")) -> ()
              n631 = global write "Robot Global Data.vi" "Reset Encoder?"(FALSE ("Reset Encoder?")) -> ()
              n632 = global write "Robot Global Data.vi" "Auto Left Drive"(0.5 ("Auto Left Drive")) -> ()
              n633 = Wait (ms)(milliseconds to wait=u32 100) -> ()  [unwired: 1 out]
              n634 = global write "Robot Global Data.vi" "Auto Right Drive"(-0.5 ("Auto Right Drive")) -> ()
            }
            frame #2 {
              # "Resets things"
              n635 = global write "Robot Global Data.vi" "Auto Right Drive"(0.0 ("Auto Right Drive")) -> ()
              n636 = global write "Robot Global Data.vi" "Auto Left Drive"(0.0 ("Auto Left Drive")) -> ()
              n637 = global write "Robot Global Data.vi" "Reset Encoder?"(TRUE ("Reset Encoder?")) -> ()
              n638 = global write "Robot Global Data.vi" "Reset Gyro?"(TRUE ("Reset Gyro?")) -> ()
              n639 = Wait (ms)(milliseconds to wait=u32 100) -> ()  [unwired: 1 out]
            }
          }
        }
      }
    }
    frame "Line Left" {
      n640 = case shown="\"R\"" w675 {
        frame "R" {
          n641 = flat-sequence {
            frame #0 {
              # "Resets things"
              n642 = global write "Robot Global Data.vi" "Auto Left Drive"(0.0 ("Auto Left Drive")) -> ()
              n643 = global write "Robot Global Data.vi" "Auto Right Drive"(0.0 ("Auto Right Drive")) -> ()
              n644 = global write "Robot Global Data.vi" "Reset Encoder?"(TRUE ("Reset Encoder?")) -> ()
              n645 = global write "Robot Global Data.vi" "Reset Gyro?"(TRUE ("Reset Gyro?")) -> ()
              n646 = Wait (ms)(milliseconds to wait=u32 100) -> ()  [unwired: 1 out]
            }
            frame #1 {
              n647 = while {
                stop <- w686 stop-if-true
                n648 = global read "Robot Global Data.vi" "EncoderValues"() -> (w691:cluster{"EncoderLeft":dbl, "EncoderRight":dbl})
                n649 = Wait (ms)(milliseconds to wait=u32 100) -> ()  [unwired: 1 out]
                n650 = call "Feet to Encoder Value.vi"("Feet"=15.5) -> ("Encoder Value"=w689:dbl)
                n651 = Unbundle(w691) -> ("EncoderLeft"=w690:dbl)  [unwired: 1 out]
                n652 = Greater Or Equal?(x=w690, y=w689) -> (x >= y?=w686:bool)
              }
              n653 = global write "Robot Global Data.vi" "Reset Gyro?"(FALSE ("Reset Gyro?")) -> ()
              n654 = global write "Robot Global Data.vi" "Reset Encoder?"(FALSE ("Reset Encoder?")) -> ()
              n655 = global write "Robot Global Data.vi" "Auto Left Drive"(0.5 ("Auto Left Drive")) -> ()
              n656 = Wait (ms)(milliseconds to wait=u32 100) -> ()  [unwired: 1 out]
              n657 = global write "Robot Global Data.vi" "Auto Right Drive"(-0.5 ("Auto Right Drive")) -> ()
            }
            frame #2 {
              # "Resets things"
              n658 = global write "Robot Global Data.vi" "Auto Right Drive"(0.0 ("Auto Right Drive")) -> ()
              n659 = global write "Robot Global Data.vi" "Auto Left Drive"(0.0 ("Auto Left Drive")) -> ()
              n660 = global write "Robot Global Data.vi" "Reset Encoder?"(TRUE ("Reset Encoder?")) -> ()
              n661 = global write "Robot Global Data.vi" "Reset Gyro?"(TRUE ("Reset Gyro?")) -> ()
              n662 = Wait (ms)(milliseconds to wait=u32 100) -> ()  [unwired: 1 out]
            }
            frame #3 {
              n663 = global write "Robot Global Data.vi" "Reset Encoder?"(TRUE ("Reset Encoder?")) -> ()
              n664 = global write "Robot Global Data.vi" "Reset Gyro?"(TRUE ("Reset Gyro?")) -> ()
              n665 = global write "Robot Global Data.vi" "Auto Left Drive"(0.7 ("Auto Left Drive")) -> ()
              n666 = global write "Robot Global Data.vi" "Auto Right Drive"(0.7 ("Auto Right Drive")) -> ()
              n667 = Wait (ms)(milliseconds to wait=u32 600) -> ()  [unwired: 1 out]
            }
            frame #4 {
              # "Resets things"
              n668 = global write "Robot Global Data.vi" "Auto Right Drive"(0.0 ("Auto Right Drive")) -> ()
              n669 = global write "Robot Global Data.vi" "Auto Left Drive"(0.0 ("Auto Left Drive")) -> ()
              n670 = global write "Robot Global Data.vi" "Reset Encoder?"(TRUE ("Reset Encoder?")) -> ()
              n671 = global write "Robot Global Data.vi" "Reset Gyro?"(TRUE ("Reset Gyro?")) -> ()
              n672 = Wait (ms)(milliseconds to wait=u32 100) -> ()  [unwired: 1 out]
            }
            frame #5 {
              n673 = while {
                stop <- w712 stop-if-true
                n674 = global read "Robot Global Data.vi" "EncoderValues"() -> (w717:cluster{"EncoderLeft":dbl, "EncoderRight":dbl})
                n675 = Wait (ms)(milliseconds to wait=u32 100) -> ()  [unwired: 1 out]
                n676 = call "Feet to Encoder Value.vi"("Feet"=12.0) -> ("Encoder Value"=w715:dbl)
                n677 = Unbundle(w717) -> ("EncoderLeft"=w716:dbl)  [unwired: 1 out]
                n678 = Greater Or Equal?(x=w716, y=w715) -> (x >= y?=w712:bool)
              }
              n679 = global write "Robot Global Data.vi" "Reset Gyro?"(FALSE ("Reset Gyro?")) -> ()
              n680 = global write "Robot Global Data.vi" "Reset Encoder?"(FALSE ("Reset Encoder?")) -> ()
              n681 = global write "Robot Global Data.vi" "Auto Left Drive"(0.5 ("Auto Left Drive")) -> ()
              n682 = Wait (ms)(milliseconds to wait=u32 100) -> ()  [unwired: 1 out]
              n683 = global write "Robot Global Data.vi" "Auto Right Drive"(-0.5 ("Auto Right Drive")) -> ()
            }
            frame #6 {
              # "Resets things"
              n684 = global write "Robot Global Data.vi" "Auto Right Drive"(0.0 ("Auto Right Drive")) -> ()
              n685 = global write "Robot Global Data.vi" "Auto Left Drive"(0.0 ("Auto Left Drive")) -> ()
              n686 = global write "Robot Global Data.vi" "Reset Encoder?"(TRUE ("Reset Encoder?")) -> ()
              n687 = global write "Robot Global Data.vi" "Reset Gyro?"(TRUE ("Reset Gyro?")) -> ()
              n688 = Wait (ms)(milliseconds to wait=u32 100) -> ()  [unwired: 1 out]
            }
            frame #7 {
              n689 = global write "Robot Global Data.vi" "Reset Encoder?"(TRUE ("Reset Encoder?")) -> ()
              n690 = global write "Robot Global Data.vi" "Reset Gyro?"(TRUE ("Reset Gyro?")) -> ()
              n691 = global write "Robot Global Data.vi" "Auto Left Drive"(1.0 ("Auto Left Drive")) -> ()
              n692 = global write "Robot Global Data.vi" "Auto Right Drive"(1.0 ("Auto Right Drive")) -> ()
              n693 = Wait (ms)(milliseconds to wait=u32 450) -> ()  [unwired: 1 out]
            }
            frame #8 {
              # "Resets things"
              n694 = global write "Robot Global Data.vi" "Auto Right Drive"(0.0 ("Auto Right Drive")) -> ()
              n695 = global write "Robot Global Data.vi" "Auto Left Drive"(0.0 ("Auto Left Drive")) -> ()
              n696 = global write "Robot Global Data.vi" "Reset Encoder?"(TRUE ("Reset Encoder?")) -> ()
              n697 = global write "Robot Global Data.vi" "Reset Gyro?"(TRUE ("Reset Gyro?")) -> ()
              n698 = Wait (ms)(milliseconds to wait=u32 100) -> ()  [unwired: 1 out]
            }
            frame #9 {
              n699 = global write "Robot Global Data.vi" "Reset Gyro?"(FALSE ("Reset Gyro?")) -> ()
              n700 = global write "Robot Global Data.vi" "Reset Encoder?"(FALSE ("Reset Encoder?")) -> ()
              n701 = global write "Robot Global Data.vi" "Auto Left Drive"(0.5 ("Auto Left Drive")) -> ()
              n702 = Wait (ms)(milliseconds to wait=u32 1500) -> ()  [unwired: 1 out]
              n703 = global write "Robot Global Data.vi" "Auto Right Drive"(-0.5 ("Auto Right Drive")) -> ()
            }
            frame #10 {
              # "Resets things"
              n704 = global write "Robot Global Data.vi" "Auto Right Drive"(0.0 ("Auto Right Drive")) -> ()
              n705 = global write "Robot Global Data.vi" "Auto Left Drive"(0.0 ("Auto Left Drive")) -> ()
              n706 = global write "Robot Global Data.vi" "Reset Encoder?"(TRUE ("Reset Encoder?")) -> ()
              n707 = global write "Robot Global Data.vi" "Reset Gyro?"(TRUE ("Reset Gyro?")) -> ()
              n708 = Wait (ms)(milliseconds to wait=u32 100) -> ()  [unwired: 1 out]
            }
            frame #11 {
              n709 = global write "Robot Global Data.vi" "Auto Right Drive"(0.0 ("Auto Right Drive")) -> ()
              n710 = global write "Robot Global Data.vi" "Auto Left Drive"(0.0 ("Auto Left Drive")) -> ()
              n711 = global write "Robot Global Data.vi" "Reset Encoder?"(TRUE ("Reset Encoder?")) -> ()
              n712 = global write "Robot Global Data.vi" "Reset Gyro?"(TRUE ("Reset Gyro?")) -> ()
              n713 = Wait (ms)(milliseconds to wait=u32 750) -> ()  [unwired: 1 out]
            }
          }
        }
        frame "L", Default {
          n714 = flat-sequence {
            frame #0 {
              # "Resets things"
              n715 = global write "Robot Global Data.vi" "Auto Left Drive"(0.0 ("Auto Left Drive")) -> ()
              n716 = global write "Robot Global Data.vi" "Auto Right Drive"(0.0 ("Auto Right Drive")) -> ()
              n717 = global write "Robot Global Data.vi" "Reset Encoder?"(TRUE ("Reset Encoder?")) -> ()
              n718 = global write "Robot Global Data.vi" "Reset Gyro?"(TRUE ("Reset Gyro?")) -> ()
              n719 = Wait (ms)(milliseconds to wait=u32 100) -> ()  [unwired: 1 out]
            }
            frame #1 {
              n720 = while {
                stop <- w758 stop-if-true
                n721 = global read "Robot Global Data.vi" "EncoderValues"() -> (w763:cluster{"EncoderLeft":dbl, "EncoderRight":dbl})
                n722 = Wait (ms)(milliseconds to wait=u32 100) -> ()  [unwired: 1 out]
                n723 = call "Feet to Encoder Value.vi"("Feet"=9.0) -> ("Encoder Value"=w761:dbl)
                n724 = Unbundle(w763) -> ("EncoderLeft"=w762:dbl)  [unwired: 1 out]
                n725 = Greater Or Equal?(x=w762, y=w761) -> (x >= y?=w758:bool)
              }
              n726 = global write "Robot Global Data.vi" "Reset Gyro?"(FALSE ("Reset Gyro?")) -> ()
              n727 = global write "Robot Global Data.vi" "Reset Encoder?"(FALSE ("Reset Encoder?")) -> ()
              n728 = global write "Robot Global Data.vi" "Auto Left Drive"(0.5 ("Auto Left Drive")) -> ()
              n729 = Wait (ms)(milliseconds to wait=u32 100) -> ()  [unwired: 1 out]
              n730 = global write "Robot Global Data.vi" "Auto Right Drive"(-0.5 ("Auto Right Drive")) -> ()
            }
            frame #2 {
              # "Resets things"
              n731 = global write "Robot Global Data.vi" "Auto Right Drive"(0.0 ("Auto Right Drive")) -> ()
              n732 = global write "Robot Global Data.vi" "Auto Left Drive"(0.0 ("Auto Left Drive")) -> ()
              n733 = global write "Robot Global Data.vi" "Reset Encoder?"(TRUE ("Reset Encoder?")) -> ()
              n734 = global write "Robot Global Data.vi" "Reset Gyro?"(TRUE ("Reset Gyro?")) -> ()
              n735 = Wait (ms)(milliseconds to wait=u32 100) -> ()  [unwired: 1 out]
            }
          }
        }
      }
    }
    frame "Test" {
    }
  }
